vi "CONTROLE_COMPLETO_2808.vi"() -> ()   [LabVIEW 2017]
panel:
  in  "stop":bool
  out "CODIGO\nPEÇA":dbl
  out "POS_FUT":dbl
  out "POS_ATUAL":dbl
  out "DEPÓSITO":bool
  out "POSICIONAMENTO":bool
  out "TRANSPORTE":bool
  out "EM ESPERA":bool
  in  "RUN":bool
  in  "SENTIDO":bool
  in  "ESTEIRA":bool
  out "MANUAL":bool
  out "AUTOMÁTICO":bool
  in  "MAN":bool
  out "COD_S4 2":dbl
  in  "TAMANHO_S4 2":enum16{"PEQUENO", "MÉDIO", "GRANDE", "DEFAULT"}(ring)
  in  "COR_S4 2":enum16{"COR 3", "COR 2", "COR 1", "DEFAULT"}(ring)
  in  "MATERIAL_S4 2":enum16{"METÁLICO", "NÃO METÁLICO", "DEFAULT"}(ring)
  out "COD_S3 2":dbl
  in  "TAMANHO_S3 2":enum16{"PEQUENO", "MÉDIO", "GRANDE", "DEFAULT"}(ring)
  in  "COR_S3 2":enum16{"COR 3", "COR 2", "COR 1", "DEFAULT"}(ring)
  in  "MATERIAL_S3 2":enum16{"METÁLICO", "NÃO METÁLICO", "DEFAULT"}(ring)
  out "COD_S2 2":dbl
  in  "TAMANHO_S2 2":enum16{"PEQUENO", "MÉDIO", "GRANDE", "DEFAULT"}(ring)
  in  "COR_S2 2":enum16{"COR 3", "COR 2", "COR 1", "DEFAULT"}(ring)
  in  "MATERIAL_S2 2":enum16{"METÁLICO", "NÃO METÁLICO", "DEFAULT"}(ring)
  out "COD_S1 2":dbl
  in  "TAMANHO_S1 2":enum16{"PEQUENO", "MÉDIO", "GRANDE", "DEFAULT"}(ring)
  in  "COR_S1 2":enum16{"COR 3", "COR 2", "COR 1", "DEFAULT"}(ring)
  in  "MATERIAL_S1 2":enum16{"METÁLICO", "NÃO METÁLICO", "DEFAULT"}(ring)
  out "CONFIGURAÇÃO CONFLITANTE 2":bool
  out "PEÇA NÃO\nCONFIGURADA":bool
  out "ESTEIRA RUN":bool
  out "PEÇA NO\nSLOT":bool
  out "MATERIAL\nMETÁLICO":bool
  out "COR_3I 2":bool
  out "COR_2I 2":bool
  out "COR_1I 2":bool
  out "TAM_PI 2":bool
  out "TAM_MI 2":bool
  out "TAM_GI 2":bool
  out "PEÇA NA\nESTEIRA":bool
  out "ESQ 2":bool
  out "DIR 2":bool
  out "RUN":bool
  out "SLOT 8":bool
  out "SLOT 7":bool
  out "SLOT 6":bool
  out "SLOT 5":bool
  out "POS_4 2":bool
  out "POS_3 2":bool
  out "POS_2 2":bool
  out "POS_1 2":bool
  out "Numeric 2":i32
  out "Numeric":i32
  in  "RESET":bool
  out "COD_CT":dbl
  out "COD_MT":dbl
  out "COD_MC":dbl
  out "COD_T":dbl
  out "COD_C":dbl
  out "COD_M":dbl
  out "2":bool
  out "4":bool
  out "3":bool
  out "1":bool
  out "CONT_1":dbl
  # "MÓDULO"
  # "UNIVERSIDADE FEDERAL DE SÃO JOÃO DEL-REI\nCAMPUS ALTO PARAOPEBA - ENGENHARIA MECATRÔNICA"
  # "2808"
  # "LABORATÓRIO DE CONTROLE E AUTOMAÇÃO"
  # "MODO"
  # "CONTROLE MANUAL"
  # "CONFIGURAÇÃO DO SISTEMA DE SELEÇÃO"
  # "SLOT 1"
  # "SLOT 2"
  # "SLOT 3"
  # "SLOT 4"
  # "POSICIONADOR"
  # "MATERIAL"
  # "RUN"
  # "COR"
  # "CONTROLE AUTOMÁTICO"
  # "TAMANHO"
  # "CÓDIGO\nSLOT"
  # "SINÓPTICO SISTEMA DE CONTROLE, SELEÇÃO E TRANSPORTE DE PEÇAS"
  # "PEÇA GRANDE"
  # "COR 1"
  # "POSIÇÃO\nATUAL"
  # "COR 2"
  # "PEÇA MÉDIA"
  # "1"
  # "2"
  # "3"
  # "4"
  # "COR 3"
  # "PEÇA PEQUENA"
  # "ESQ"
  # "MOTOR POSICIONADOR"
  # "DIR"
  # "MOTOR\nESTEIRA"
  # "POSIÇÃO\nFUTURA"
  # "1"
  # "2"
  # "4"
  # "3"
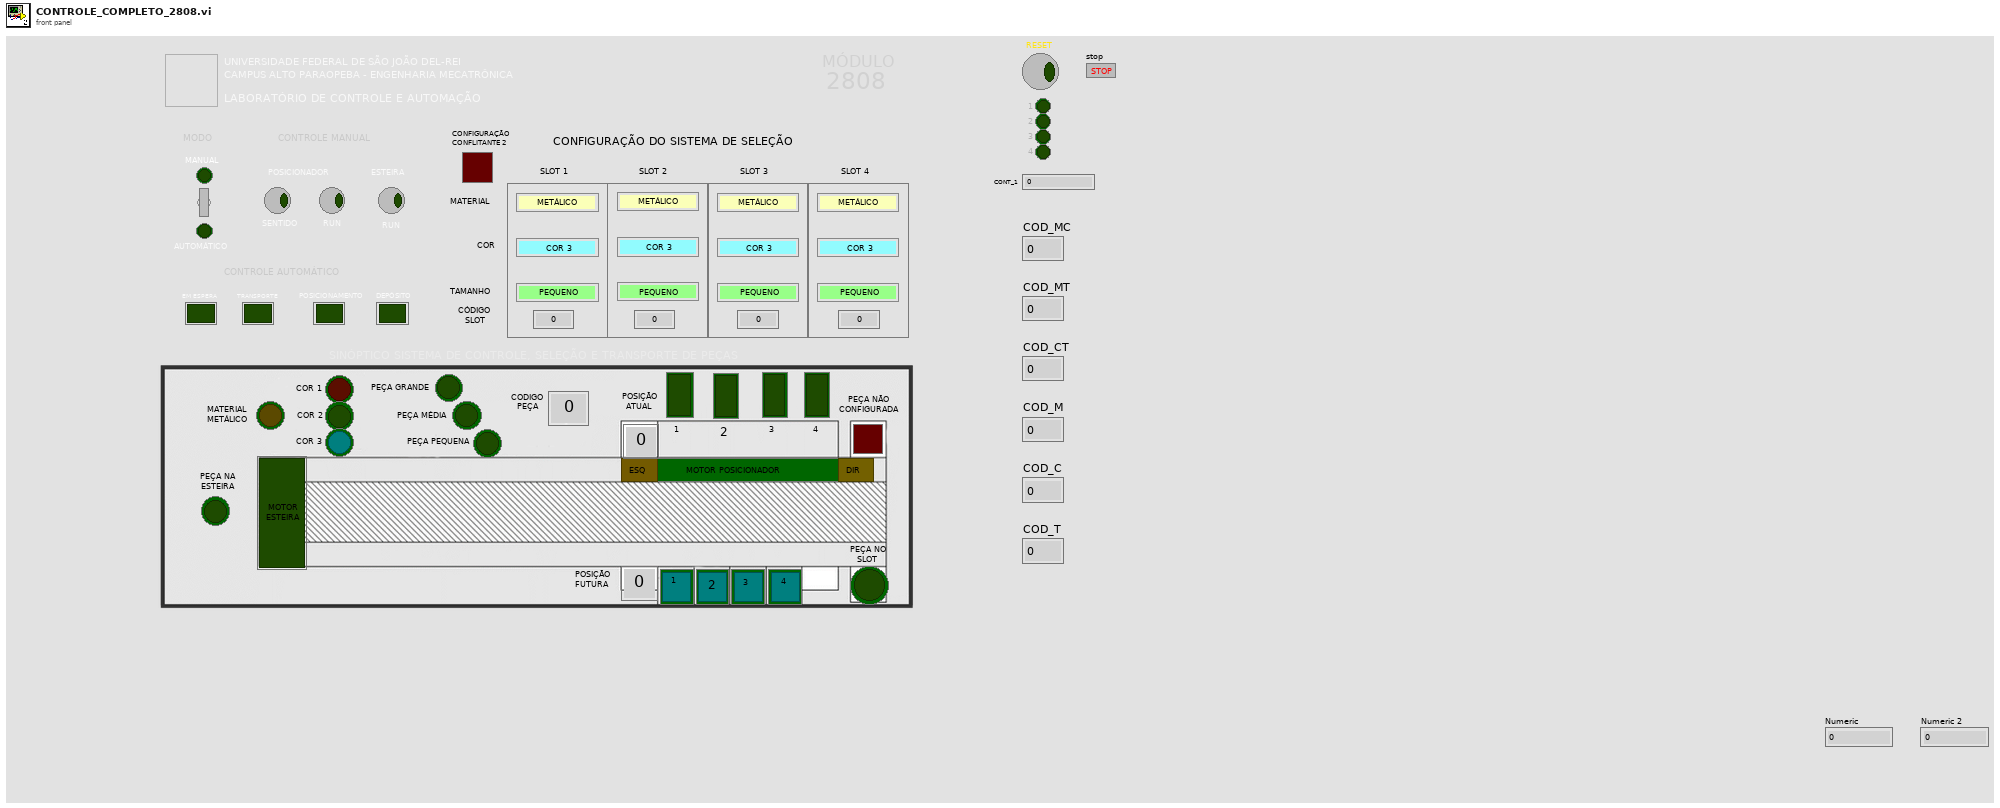
[diagram p1: front panel]
types:
  T1 = enum16{"DEPOSITO HASTE", "POSICIONAMENTO HASTE", "AQUISIÇÃO DE DADOS", "EM ESPERA"}
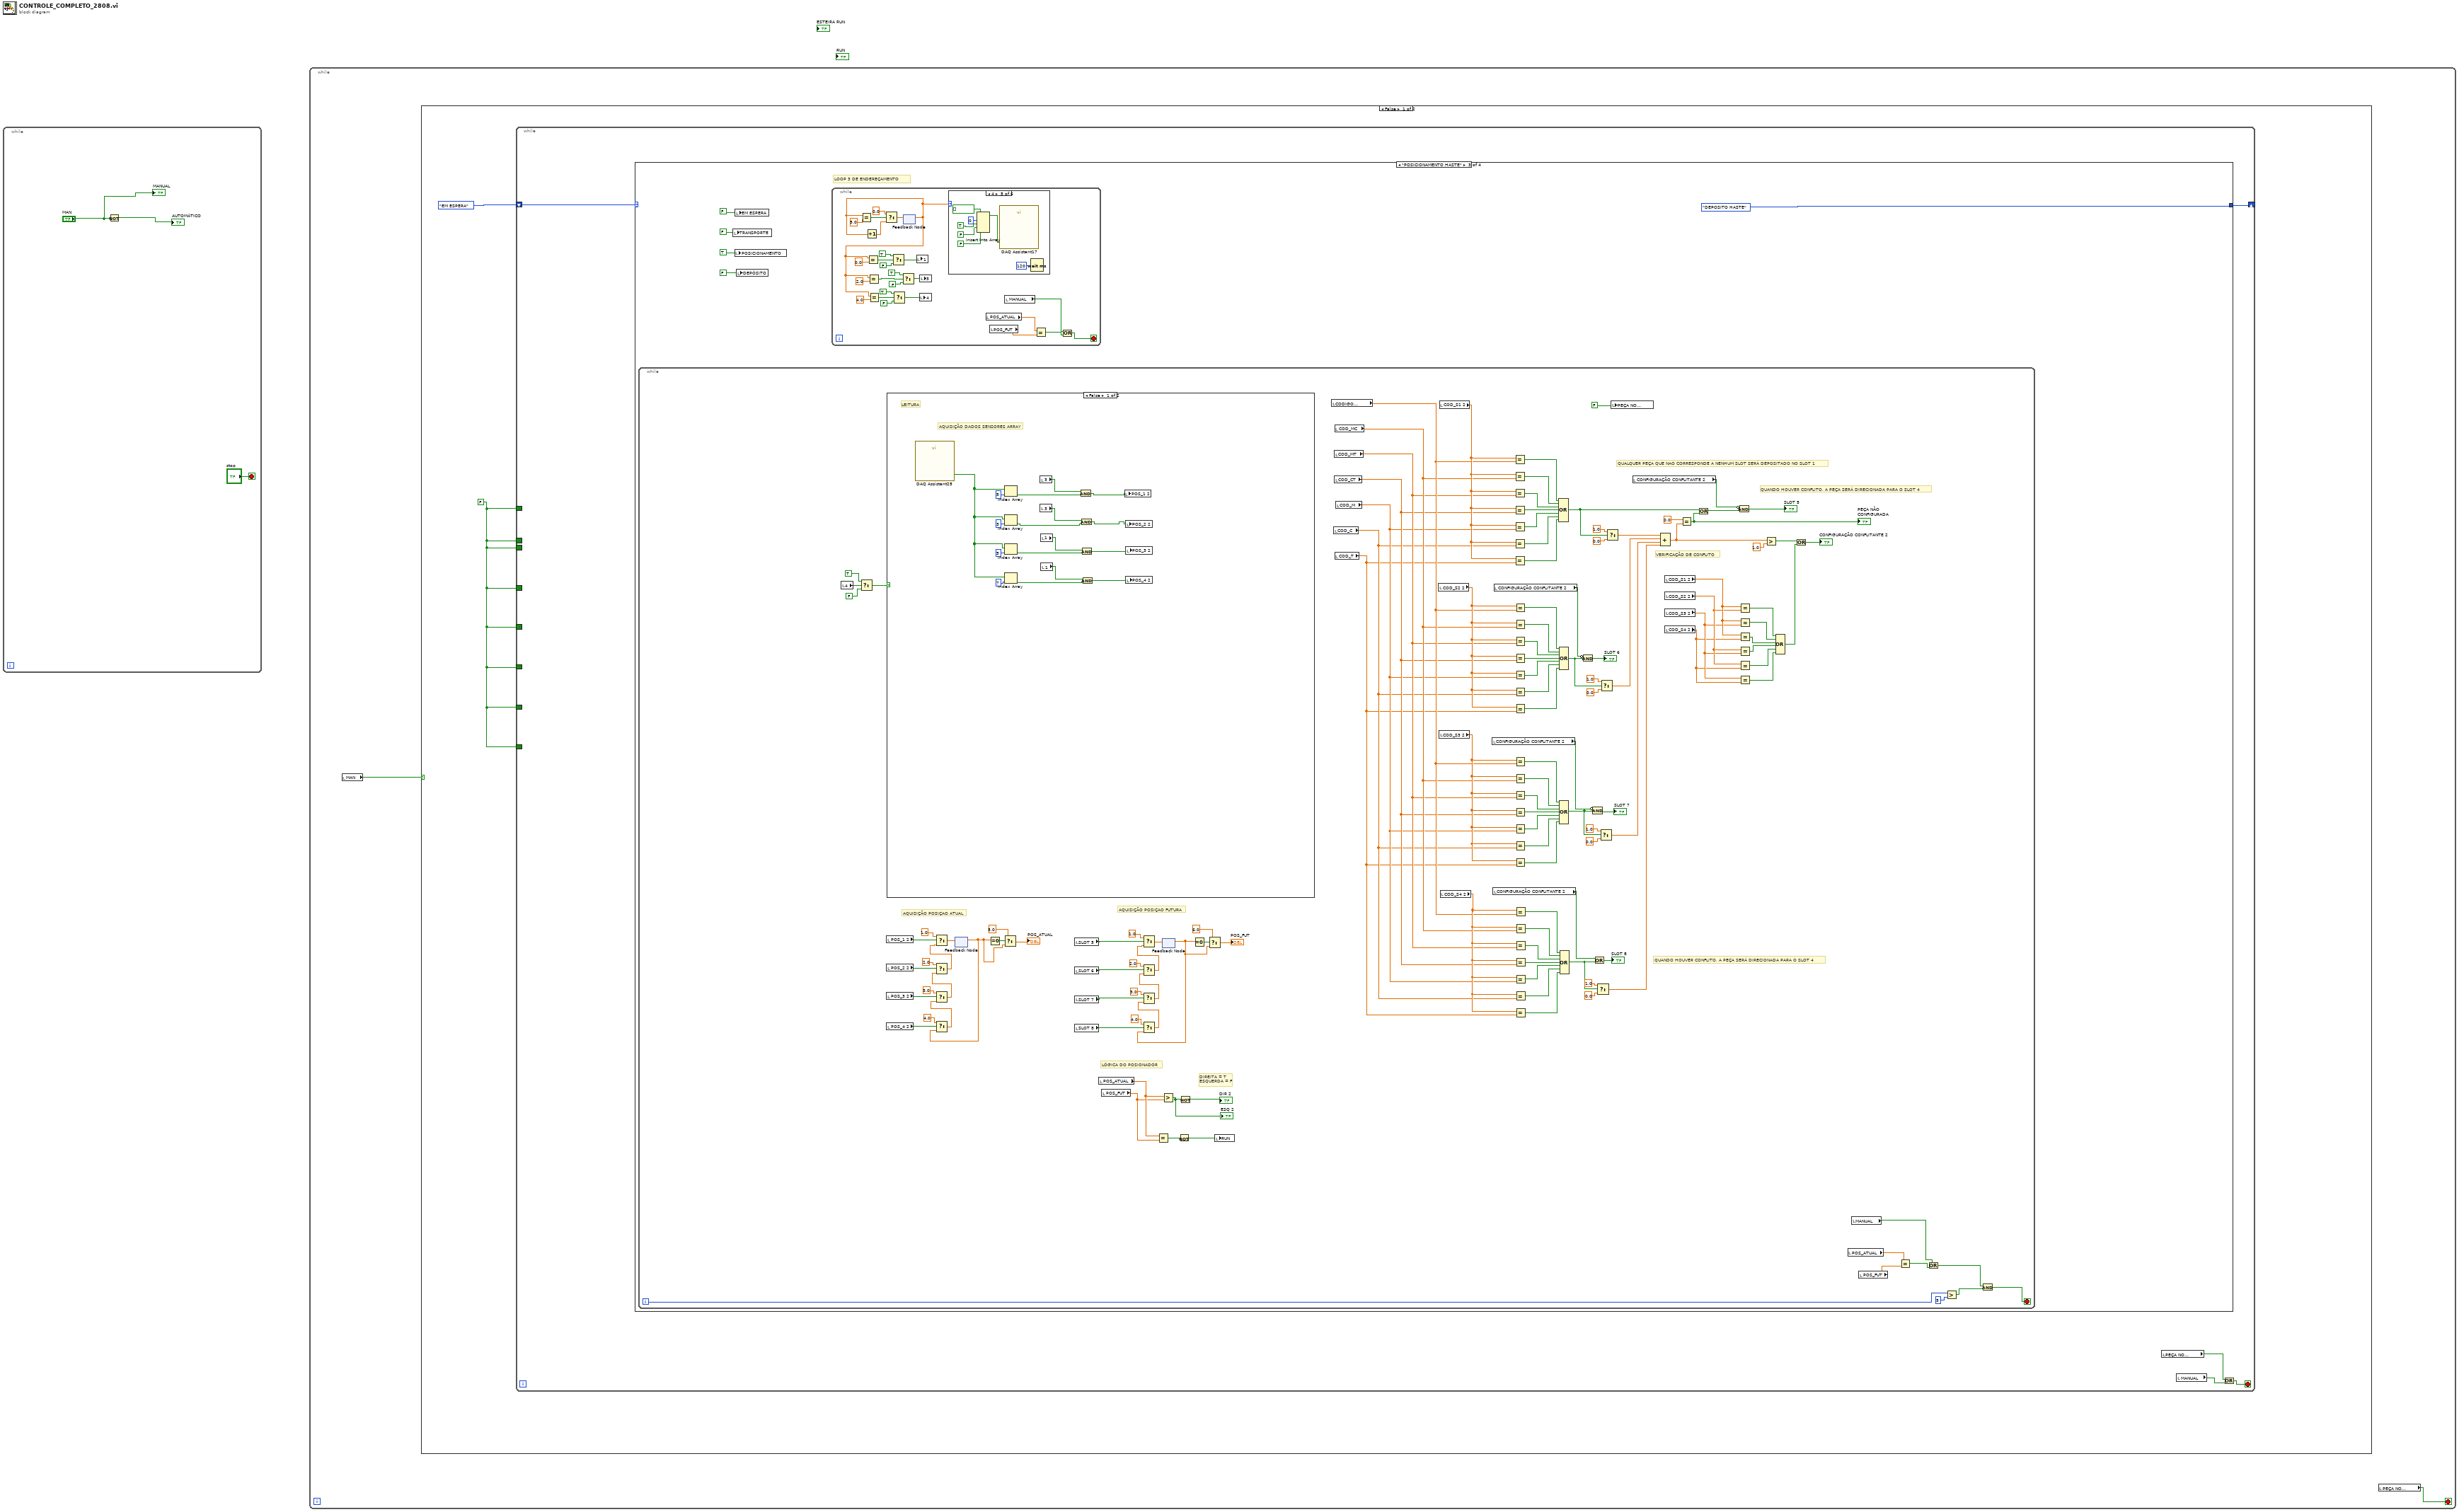
[diagram p0: block diagram]
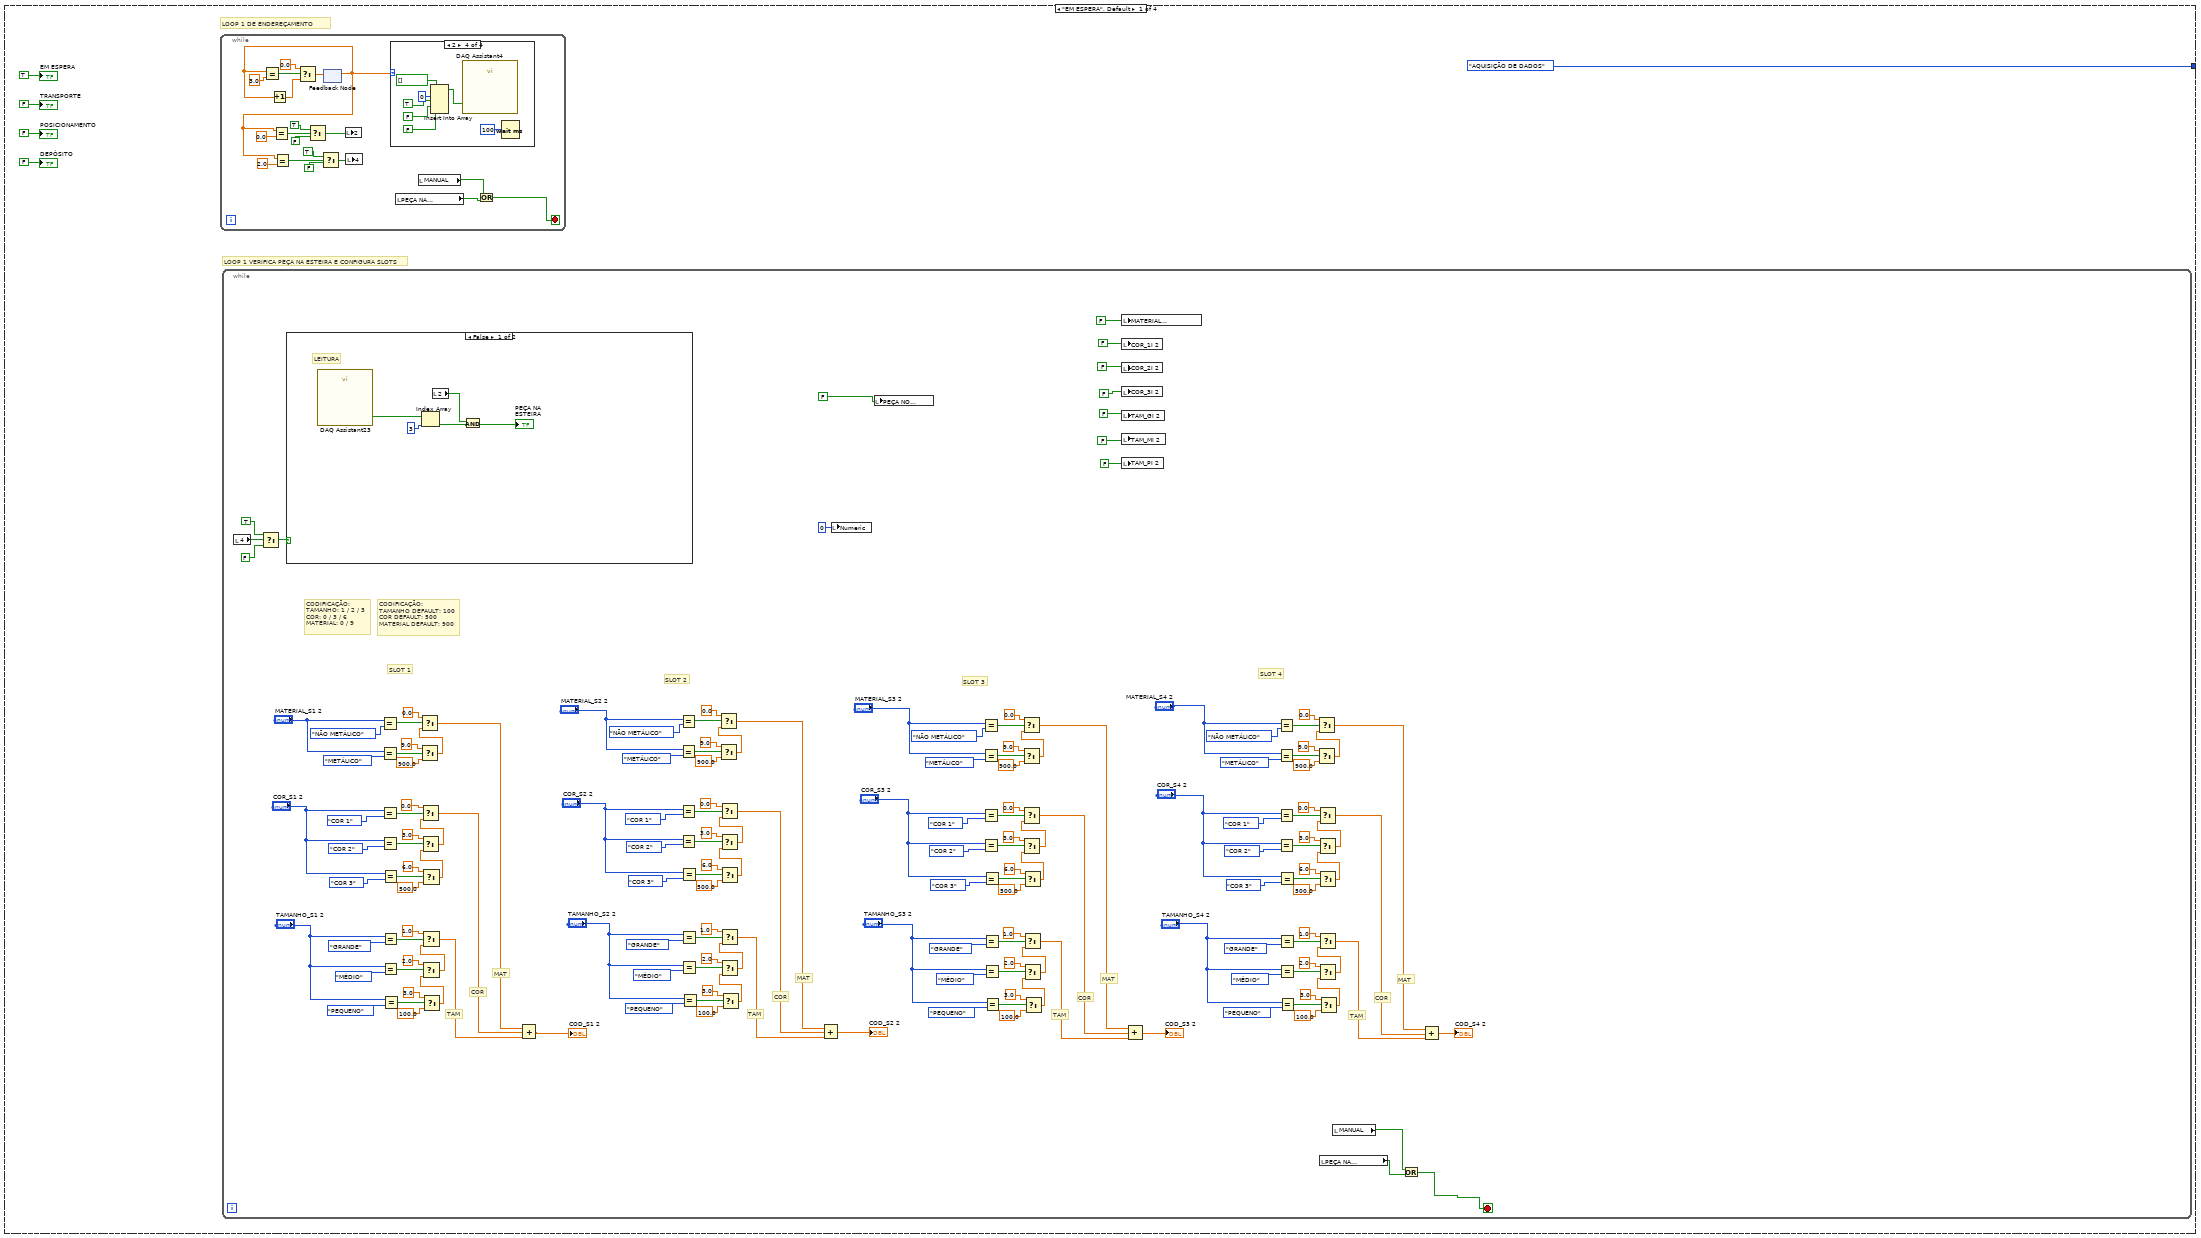
[diagram p2: hidden frame]
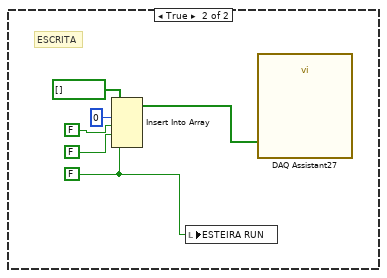
[diagram p3: hidden frame]
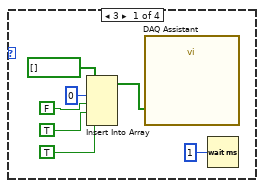
[diagram p4: hidden frame]
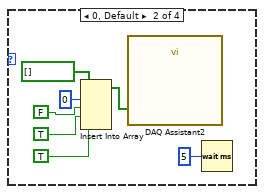
[diagram p5: hidden frame]
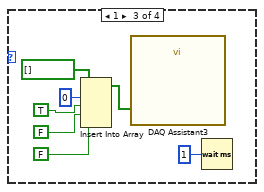
[diagram p6: hidden frame]
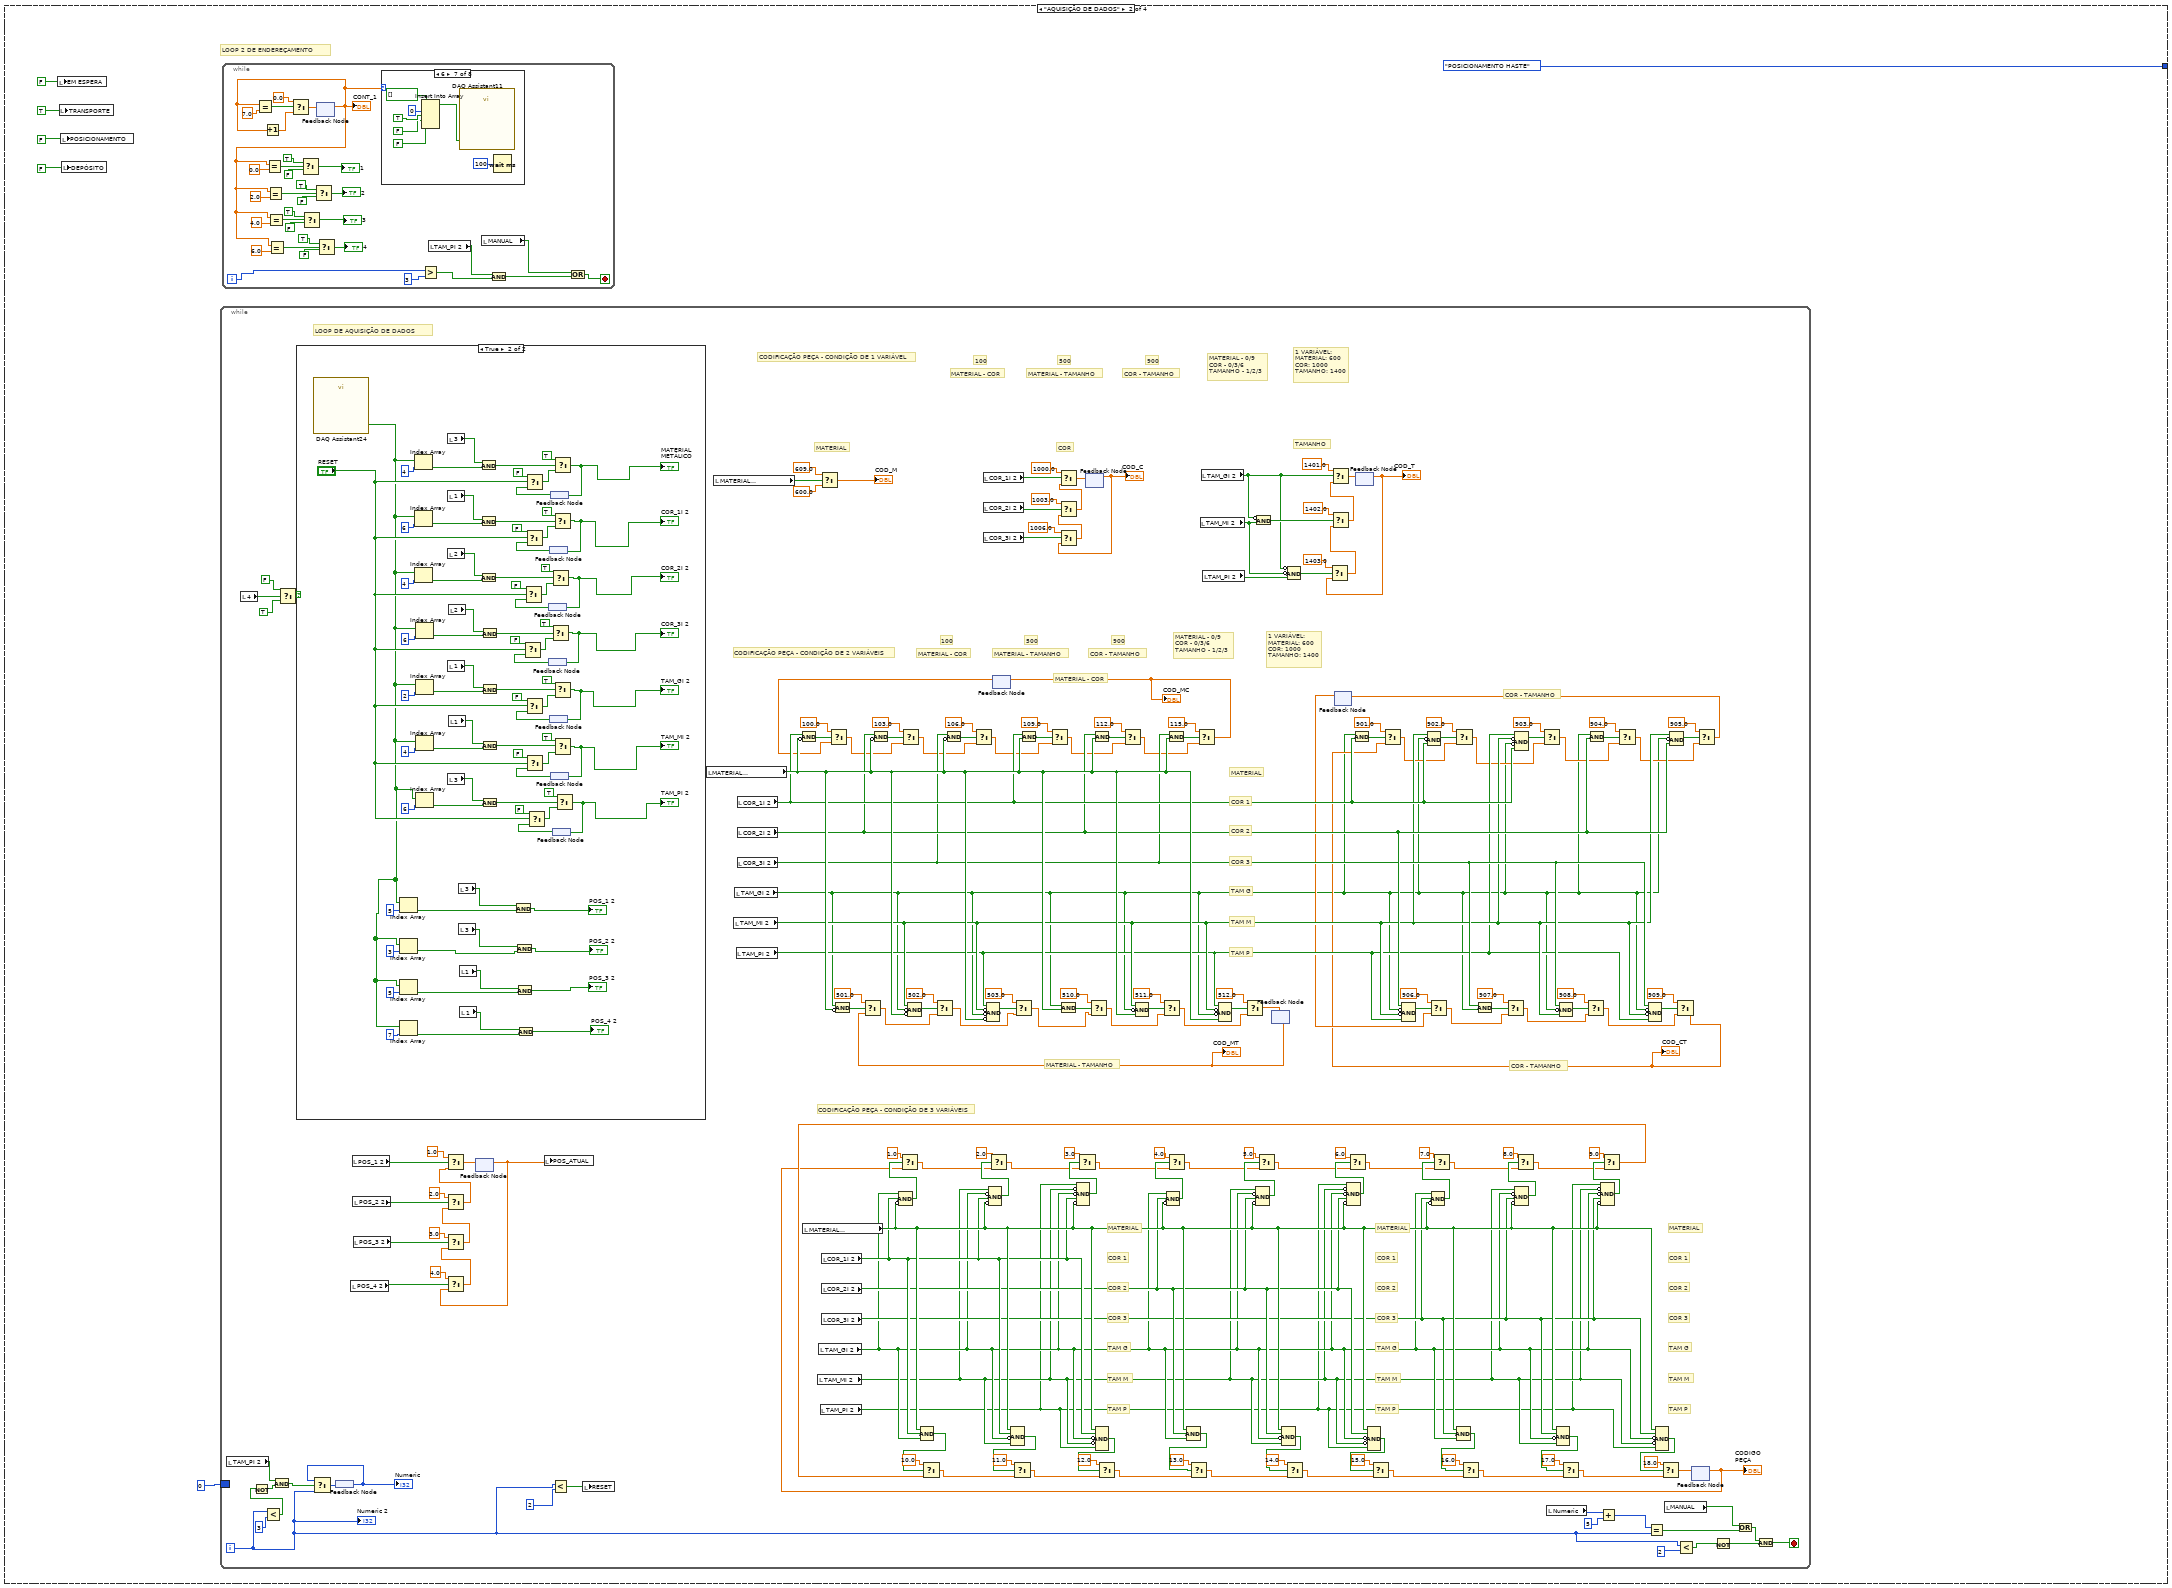
[diagram p7: hidden frame]
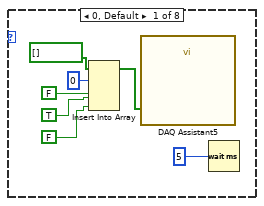
[diagram p8: hidden frame]
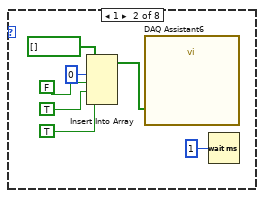
[diagram p9: hidden frame]
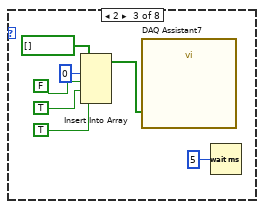
[diagram p10: hidden frame]
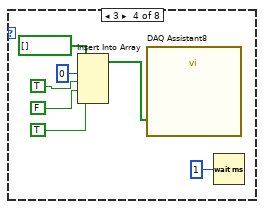
[diagram p11: hidden frame]
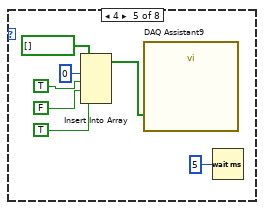
[diagram p12: hidden frame]
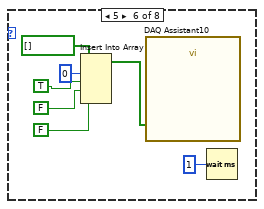
[diagram p13: hidden frame]
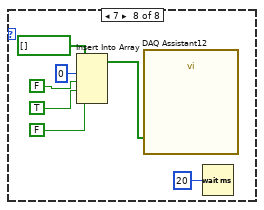
[diagram p14: hidden frame]
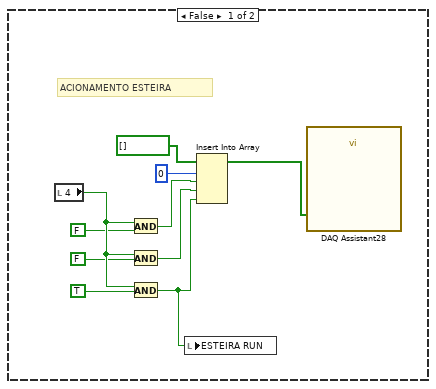
[diagram p15: hidden frame]
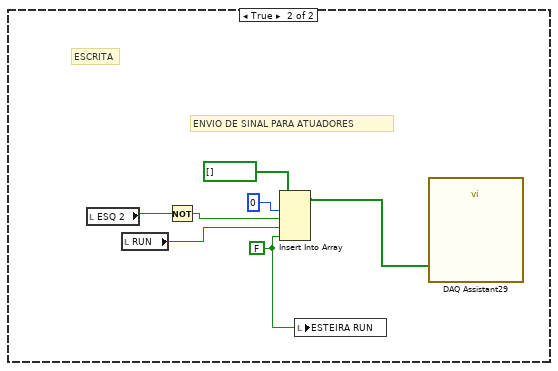
[diagram p16: hidden frame]
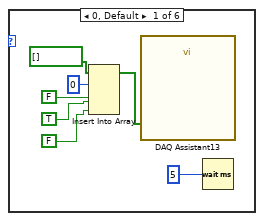
[diagram p17: hidden frame]
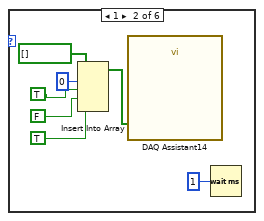
[diagram p18: hidden frame]
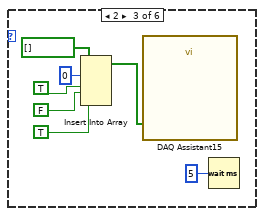
[diagram p19: hidden frame]
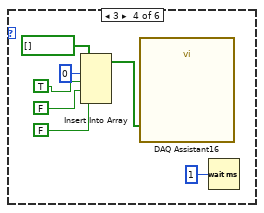
[diagram p20: hidden frame]
diagram:
  n1 = while {
    stop <- "stop" stop-if-true
    n2 = Not(x="MAN") -> (.not. x?=→"AUTOMÁTICO":bool)
    "MANUAL" <- "MAN"
  }
  n3 = while {
    stop <- w4 stop-if-true
    n4 = local read "MAN"() -> (w5:bool)
    n5 = case shown="False" w5 {
      frame False {
        w6 = FALSE
        n6 = while {
          shift-right: [w11] -> _
          shift-left: T1."EM ESPERA" -> [w12]
          border: w6 -> [_]
          border: w6 -> [_]
          border: w6 -> [_]
          border: w6 -> [_]
          border: w6 -> [_]
          border: w6 -> [_]
          border: w6 -> [_]
          border: w6 -> [_]
          stop <- w8 stop-if-true
          n7 = case shown="\"POSICIONAMENTO HASTE\"" w12 {
            tunnel: [T1."AQUISIÇÃO DE DADOS" T1."POSICIONAMENTO HASTE" T1."DEPOSITO HASTE" T1."EM ESPERA"] -> w11
            frame "EM ESPERA", Default {
              # "LOOP 1 VERIFICA PEÇA NA ESTEIRA E CONFIGURA SLOTS"
              # "LOOP 1 DE ENDEREÇAMENTO"
              n8 = while {
                stop <- w201 stop-if-true
                n9 = feedback #1() -> (w206:dbl)  [unwired: 1 in]
                n10 = Equal?(x=w206, y=3.0) -> (x = y?=w219:bool)
                n11 = Increment(x=w206) -> (x+1=w216:dbl)
                n12 = Equal?(x=w206, y=0.0) -> (x = y?=w212:bool)
                n13 = Equal?(x=w206, y=2.0) -> (x = y?=w207:bool)
                n14 = Select(t=0.0, s=w219, f=w216) -> (s? t:f=w218:dbl)
                n15 = Select(t=TRUE, s=w212, f=FALSE) -> (s? t:f=w205:bool)
                n16 = Select(t=TRUE, s=w207, f=FALSE) -> (s? t:f=w204:bool)
                n17 = feedback-in #1(w218) -> ()
                n18 = local write "2"(w205) -> ()
                n19 = local write "4"(w204) -> ()
                n20 = case shown="2" w206 {
                  frame 3 {
                    n21 = Insert Into Array(array=bool[] [], index=0, new element #1=FALSE, new element #2=TRUE, new element #3=TRUE) -> (w220:bool[])
                    n22 = call "DAQ Assistant"("data"=w220) -> ()  [unwired: 17 in, 2 out]
                    n23 = Wait (ms)(milliseconds to wait=u32 1) -> ()  [unwired: 1 out]
                  }
                  frame 0, Default {
                    n24 = Insert Into Array(array=bool[] [], index=0, new element #1=FALSE, new element #2=TRUE, new element #3=TRUE) -> (w227:bool[])
                    n25 = call "DAQ Assistant2"("data"=w227) -> ()  [unwired: 17 in, 2 out]
                    n26 = Wait (ms)(milliseconds to wait=u32 5) -> ()  [unwired: 1 out]
                  }
                  frame 1 {
                    n27 = Insert Into Array(array=bool[] [], index=0, new element #1=TRUE, new element #2=FALSE, new element #3=FALSE) -> (w234:bool[])
                    n28 = call "DAQ Assistant3"("data"=w234) -> ()  [unwired: 17 in, 2 out]
                    n29 = Wait (ms)(milliseconds to wait=u32 1) -> ()  [unwired: 1 out]
                  }
                  frame 2 {
                    n30 = Insert Into Array(array=bool[] [], index=0, new element #1=TRUE, new element #2=FALSE, new element #3=FALSE) -> (w241:bool[])
                    n31 = call "DAQ Assistant4"("data"=w241) -> ()  [unwired: 17 in, 2 out]
                    n32 = Wait (ms)(milliseconds to wait=u32 100) -> ()  [unwired: 1 out]
                  }
                }
                n33 = local read "PEÇA NA\nESTEIRA"() -> (w203:bool)
                n34 = local read "MANUAL"() -> (w202:bool)
                n35 = Or(x=w202, y=w203) -> (x .or. y?=w201:bool)
              }
              n36 = while {
                stop <- w42 stop-if-true
                # "COR"
                # "MAT"
                # "TAM"
                # "COR"
                # "MAT"
                # "TAM"
                # "COR"
                # "MAT"
                # "TAM"
                # "TAM"
                # "COR"
                # "MAT"
                # "CODIFICAÇÃO:\nTAMANHO DEFAULT: 100\nCOR DEFAULT: 500\nMATERIAL DEFAULT: 900"
                # "CODIFICAÇÃO:\nTAMANHO: 1 / 2 / 3\nCOR: 0 / 3 / 6\nMATERIAL: 0 / 9"
                # "SLOT 4"
                # "SLOT 3"
                # "SLOT 2"
                # "SLOT 1"
                n37 = local read "4"() -> (w189:bool)
                n38 = Select(t=TRUE, s=w189, f=FALSE) -> (s? t:f=w186:bool)
                n39 = case shown="False" w186 {
                  frame False {
                    # "LEITURA"
                    n40 = call "DAQ Assistant23"() -> ("data"=w191:bool[])  [unwired: 17 in, 2 out]
                    n41 = Index Array(array=w191, index=3) -> (element=w192:bool)
                    n42 = local read "2"() -> (w194:bool)
                    n43 = And(x=w194, y=w192) -> (x .and. y?=→"PEÇA NA\nESTEIRA":bool)
                  }
                  frame True {
                    w196 = FALSE
                    # "ESCRITA"
                    n44 = Insert Into Array(array=bool[] [], index=0, new element #1=FALSE, new element #2=FALSE, new element #3=w196) -> (w195:bool[])
                    n45 = local write "ESTEIRA RUN"(w196) -> ()
                    n46 = call "DAQ Assistant27"("data"=w195) -> ()  [unwired: 17 in, 2 out]
                  }
                }
                n47 = Equal?(x="MATERIAL_S1 2", y=enum16{"METÁLICO", "NÃO METÁLICO", "DEFAULT"}."NÃO METÁLICO") -> (x = y?=w185:bool)
                n48 = Equal?(x="MATERIAL_S1 2", y=enum16{"METÁLICO", "NÃO METÁLICO", "DEFAULT"}."METÁLICO") -> (x = y?=w181:bool)
                n49 = Equal?(x="COR_S1 2", y=enum16{"COR 3", "COR 2", "COR 1", "DEFAULT"}."COR 1") -> (x = y?=w177:bool)
                n50 = Equal?(x="COR_S1 2", y=enum16{"COR 3", "COR 2", "COR 1", "DEFAULT"}."COR 2") -> (x = y?=w176:bool)
                n51 = Equal?(x="COR_S1 2", y=enum16{"COR 3", "COR 2", "COR 1", "DEFAULT"}."COR 3") -> (x = y?=w175:bool)
                n52 = Equal?(x="TAMANHO_S1 2", y=enum16{"PEQUENO", "MÉDIO", "GRANDE", "DEFAULT"}."GRANDE") -> (x = y?=w165:bool)
                n53 = Equal?(x="TAMANHO_S1 2", y=enum16{"PEQUENO", "MÉDIO", "GRANDE", "DEFAULT"}."MÉDIO") -> (x = y?=w164:bool)
                n54 = Equal?(x="TAMANHO_S1 2", y=enum16{"PEQUENO", "MÉDIO", "GRANDE", "DEFAULT"}."PEQUENO") -> (x = y?=w163:bool)
                n55 = Select(t=9.0, s=w181, f=900.0) -> (s? t:f=w178:dbl)
                n56 = Select(t=0.0, s=w185, f=w178) -> (s? t:f=w57:dbl)
                n57 = Select(t=6.0, s=w175, f=500.0) -> (s? t:f=w167:dbl)
                n58 = Select(t=3.0, s=w176, f=w167) -> (s? t:f=w166:dbl)
                n59 = Select(t=0.0, s=w177, f=w166) -> (s? t:f=w56:dbl)
                n60 = Select(t=3.0, s=w163, f=100.0) -> (s? t:f=w158:dbl)
                n61 = Select(t=2.0, s=w164, f=w158) -> (s? t:f=w157:dbl)
                n62 = Select(t=1.0, s=w165, f=w157) -> (s? t:f=w55:dbl)
                n63 = Compound Arithmetic op=ADD(w57, w56, w55) -> (→"COD_S1 2":dbl)
                n64 = Equal?(x="MATERIAL_S2 2", y=enum16{"METÁLICO", "NÃO METÁLICO", "DEFAULT"}."NÃO METÁLICO") -> (x = y?=w153:bool)
                n65 = Equal?(x="MATERIAL_S2 2", y=enum16{"METÁLICO", "NÃO METÁLICO", "DEFAULT"}."METÁLICO") -> (x = y?=w149:bool)
                n66 = Equal?(x="COR_S2 2", y=enum16{"COR 3", "COR 2", "COR 1", "DEFAULT"}."COR 1") -> (x = y?=w145:bool)
                n67 = Equal?(x="COR_S2 2", y=enum16{"COR 3", "COR 2", "COR 1", "DEFAULT"}."COR 2") -> (x = y?=w144:bool)
                n68 = Equal?(x="COR_S2 2", y=enum16{"COR 3", "COR 2", "COR 1", "DEFAULT"}."COR 3") -> (x = y?=w143:bool)
                n69 = Equal?(x="TAMANHO_S2 2", y=enum16{"PEQUENO", "MÉDIO", "GRANDE", "DEFAULT"}."GRANDE") -> (x = y?=w133:bool)
                n70 = Equal?(x="TAMANHO_S2 2", y=enum16{"PEQUENO", "MÉDIO", "GRANDE", "DEFAULT"}."MÉDIO") -> (x = y?=w132:bool)
                n71 = Equal?(x="TAMANHO_S2 2", y=enum16{"PEQUENO", "MÉDIO", "GRANDE", "DEFAULT"}."PEQUENO") -> (x = y?=w131:bool)
                n72 = Select(t=9.0, s=w149, f=900.0) -> (s? t:f=w146:dbl)
                n73 = Select(t=0.0, s=w153, f=w146) -> (s? t:f=w52:dbl)
                n74 = Select(t=6.0, s=w143, f=500.0) -> (s? t:f=w135:dbl)
                n75 = Select(t=3.0, s=w144, f=w135) -> (s? t:f=w134:dbl)
                n76 = Select(t=0.0, s=w145, f=w134) -> (s? t:f=w53:dbl)
                n77 = Select(t=3.0, s=w131, f=100.0) -> (s? t:f=w126:dbl)
                n78 = Select(t=2.0, s=w132, f=w126) -> (s? t:f=w125:dbl)
                n79 = Select(t=1.0, s=w133, f=w125) -> (s? t:f=w54:dbl)
                n80 = Compound Arithmetic op=ADD(w52, w53, w54) -> (→"COD_S2 2":dbl)
                n81 = local write "Numeric"(0 ("Numeric")) -> ()
                n82 = local write "PEÇA NO\nSLOT"(FALSE ("PDS_I")) -> ()
                n83 = Equal?(x="MATERIAL_S3 2", y=enum16{"METÁLICO", "NÃO METÁLICO", "DEFAULT"}."NÃO METÁLICO") -> (x = y?=w121:bool)
                n84 = Equal?(x="MATERIAL_S3 2", y=enum16{"METÁLICO", "NÃO METÁLICO", "DEFAULT"}."METÁLICO") -> (x = y?=w117:bool)
                n85 = Equal?(x="COR_S3 2", y=enum16{"COR 3", "COR 2", "COR 1", "DEFAULT"}."COR 1") -> (x = y?=w113:bool)
                n86 = Equal?(x="COR_S3 2", y=enum16{"COR 3", "COR 2", "COR 1", "DEFAULT"}."COR 2") -> (x = y?=w112:bool)
                n87 = Equal?(x="COR_S3 2", y=enum16{"COR 3", "COR 2", "COR 1", "DEFAULT"}."COR 3") -> (x = y?=w111:bool)
                n88 = Equal?(x="TAMANHO_S3 2", y=enum16{"PEQUENO", "MÉDIO", "GRANDE", "DEFAULT"}."GRANDE") -> (x = y?=w101:bool)
                n89 = Equal?(x="TAMANHO_S3 2", y=enum16{"PEQUENO", "MÉDIO", "GRANDE", "DEFAULT"}."MÉDIO") -> (x = y?=w100:bool)
                n90 = Equal?(x="TAMANHO_S3 2", y=enum16{"PEQUENO", "MÉDIO", "GRANDE", "DEFAULT"}."PEQUENO") -> (x = y?=w99:bool)
                n91 = Select(t=9.0, s=w117, f=900.0) -> (s? t:f=w114:dbl)
                n92 = Select(t=0.0, s=w121, f=w114) -> (s? t:f=w49:dbl)
                n93 = Select(t=6.0, s=w111, f=500.0) -> (s? t:f=w103:dbl)
                n94 = Select(t=3.0, s=w112, f=w103) -> (s? t:f=w102:dbl)
                n95 = Select(t=0.0, s=w113, f=w102) -> (s? t:f=w50:dbl)
                n96 = Select(t=3.0, s=w99, f=100.0) -> (s? t:f=w94:dbl)
                n97 = Select(t=2.0, s=w100, f=w94) -> (s? t:f=w93:dbl)
                n98 = Select(t=1.0, s=w101, f=w93) -> (s? t:f=w51:dbl)
                n99 = local write "MATERIAL\nMETÁLICO"(FALSE) -> ()
                n100 = local write "COR_1I 2"(FALSE) -> ()
                n101 = local write "COR_2I 2"(FALSE) -> ()
                n102 = local write "COR_3I 2"(FALSE) -> ()
                n103 = local write "TAM_GI 2"(FALSE) -> ()
                n104 = local write "TAM_MI 2"(FALSE) -> ()
                n105 = local write "TAM_PI 2"(FALSE) -> ()
                n106 = Compound Arithmetic op=ADD(w49, w50, w51) -> (→"COD_S3 2":dbl)
                n107 = Equal?(x="MATERIAL_S4 2", y=enum16{"METÁLICO", "NÃO METÁLICO", "DEFAULT"}."NÃO METÁLICO") -> (x = y?=w89:bool)
                n108 = Equal?(x="MATERIAL_S4 2", y=enum16{"METÁLICO", "NÃO METÁLICO", "DEFAULT"}."METÁLICO") -> (x = y?=w85:bool)
                n109 = Equal?(x="COR_S4 2", y=enum16{"COR 3", "COR 2", "COR 1", "DEFAULT"}."COR 1") -> (x = y?=w81:bool)
                n110 = Equal?(x="COR_S4 2", y=enum16{"COR 3", "COR 2", "COR 1", "DEFAULT"}."COR 2") -> (x = y?=w80:bool)
                n111 = Equal?(x="COR_S4 2", y=enum16{"COR 3", "COR 2", "COR 1", "DEFAULT"}."COR 3") -> (x = y?=w79:bool)
                n112 = Equal?(x="TAMANHO_S4 2", y=enum16{"PEQUENO", "MÉDIO", "GRANDE", "DEFAULT"}."GRANDE") -> (x = y?=w69:bool)
                n113 = Equal?(x="TAMANHO_S4 2", y=enum16{"PEQUENO", "MÉDIO", "GRANDE", "DEFAULT"}."MÉDIO") -> (x = y?=w68:bool)
                n114 = Equal?(x="TAMANHO_S4 2", y=enum16{"PEQUENO", "MÉDIO", "GRANDE", "DEFAULT"}."PEQUENO") -> (x = y?=w67:bool)
                n115 = Select(t=9.0, s=w85, f=900.0) -> (s? t:f=w82:dbl)
                n116 = Select(t=0.0, s=w89, f=w82) -> (s? t:f=w46:dbl)
                n117 = Select(t=6.0, s=w79, f=500.0) -> (s? t:f=w71:dbl)
                n118 = Select(t=3.0, s=w80, f=w71) -> (s? t:f=w70:dbl)
                n119 = Select(t=0.0, s=w81, f=w70) -> (s? t:f=w47:dbl)
                n120 = Select(t=3.0, s=w67, f=100.0) -> (s? t:f=w62:dbl)
                n121 = Select(t=2.0, s=w68, f=w62) -> (s? t:f=w61:dbl)
                n122 = Select(t=1.0, s=w69, f=w61) -> (s? t:f=w48:dbl)
                n123 = local read "PEÇA NA\nESTEIRA"() -> (w45:bool)
                n124 = local read "MANUAL"() -> (w44:bool)
                n125 = Or(x=w44, y=w45) -> (x .or. y?=w42:bool)
                n126 = Compound Arithmetic op=ADD(w46, w47, w48) -> (→"COD_S4 2":dbl)
              }
              "TRANSPORTE" <- FALSE
              "POSICIONAMENTO" <- FALSE
              "DEPÓSITO" <- FALSE
              "EM ESPERA" <- TRUE
            }
            frame "AQUISIÇÃO DE DADOS" {
              # "LOOP 2 DE ENDEREÇAMENTO"
              n127 = local write "EM ESPERA"(FALSE) -> ()
              n128 = local write "TRANSPORTE"(TRUE) -> ()
              n129 = local write "POSICIONAMENTO"(FALSE) -> ()
              n130 = local write "DEPÓSITO"(FALSE) -> ()
              n131 = while {
                border: 0 -> [_]
                i -> [w348]
                stop <- w352 stop-if-true
                # "CODIFICAÇÃO PEÇA - CONDIÇÃO DE 3 VARIÁVEIS"
                # "TAM P"
                # "TAM M"
                # "TAM G"
                # "COR 3"
                # "COR 2"
                # "COR 1"
                # "MATERIAL"
                # "TAM P"
                # "TAM M"
                # "TAM G"
                # "COR 3"
                # "COR 2"
                # "COR 1"
                # "MATERIAL"
                # "TAM P"
                # "TAM M"
                # "TAM G"
                # "COR 3"
                # "COR 2"
                # "COR 1"
                # "MATERIAL"
                # "1 VARIÁVEL:\nMATERIAL: 600\nCOR: 1000\nTAMANHO: 1400"
                # "COR - TAMANHO"
                # "COR - TAMANHO"
                # "MATERIAL - TAMANHO"
                # "MATERIAL - COR"
                # "MATERIAL - 0/9\nCOR - 0/3/6\nTAMANHO - 1/2/3"
                # "900"
                # "500"
                # "100"
                # "COR - TAMANHO"
                # "MATERIAL - TAMANHO"
                # "MATERIAL - COR"
                # "CODIFICAÇÃO PEÇA - CONDIÇÃO DE 2 VARIÁVEIS"
                # "TAM P"
                # "TAM M"
                # "TAM G"
                # "COR 3"
                # "COR 2"
                # "COR 1"
                # "MATERIAL"
                # "TAMANHO"
                # "COR"
                # "1 VARIÁVEL:\nMATERIAL: 600\nCOR: 1000\nTAMANHO: 1400"
                # "MATERIAL"
                # "MATERIAL - 0/9\nCOR - 0/3/6\nTAMANHO - 1/2/3"
                # "900"
                # "500"
                # "100"
                # "COR - TAMANHO"
                # "MATERIAL - TAMANHO"
                # "MATERIAL - COR"
                # "CODIFICAÇÃO PEÇA - CONDIÇÃO DE 1 VARIÁVEL"
                # "LOOP DE AQUISIÇÃO DE DADOS"
                n132 = local read "TAM_PI 2"() -> (w344:bool)
                n133 = local read "4"() -> (w540:bool)
                n134 = Less?(x=w348, y=3) -> (x < y?=w345:bool)
                n135 = Not(x=w345) -> (.not. x?=w346:bool)
                n136 = And(x=w344, y=w346) -> (x .and. y?=w343:bool)
                n137 = Select(t=FALSE, s=w540, f=TRUE) -> (s? t:f=w539:bool)
                n138 = case shown="True" w539 {
                  frame False {
                    # "ACIONAMENTO ESTEIRA"
                    n139 = local read "4"() -> (w550:bool)
                    n140 = And(x=w550, y=FALSE) -> (x .and. y?=w549:bool)
                    n141 = And(x=w550, y=FALSE) -> (x .and. y?=w548:bool)
                    n142 = And(x=w550, y=TRUE) -> (x .and. y?=w542:bool)
                    n143 = local write "ESTEIRA RUN"(w542) -> ()
                    n144 = Insert Into Array(array=bool[] [], index=0, new element #1=w549, new element #2=w548, new element #3=w542) -> (w541:bool[])
                    n145 = call "DAQ Assistant28"("data"=w541) -> ()  [unwired: 17 in, 2 out]
                  }
                  frame True {
                    n146 = call "DAQ Assistant24"() -> ("data"=w562:bool[])  [unwired: 17 in, 2 out]
                    n147 = Index Array(array=w562, index=5) -> (element=w566:bool)
                    n148 = Index Array(array=w562, index=3) -> (element=w565:bool)
                    n149 = Index Array(array=w562, index=5) -> (element=w564:bool)
                    n150 = Index Array(array=w562, index=7) -> (element=w563:bool)
                    n151 = Index Array(array=w562, index=4) -> (element=w577:bool)
                    n152 = Index Array(array=w562, index=6) -> (element=w576:bool)
                    n153 = Index Array(array=w562, index=4) -> (element=w575:bool)
                    n154 = Index Array(array=w562, index=6) -> (element=w574:bool)
                    n155 = Index Array(array=w562, index=2) -> (element=w573:bool)
                    n156 = Index Array(array=w562, index=4) -> (element=w572:bool)
                    n157 = Index Array(array=w562, index=6) -> (element=w571:bool)
                    n158 = local read "3"() -> (w596:bool)
                    n159 = local read "1"() -> (w595:bool)
                    n160 = local read "2"() -> (w594:bool)
                    n161 = local read "1"() -> (w592:bool)
                    n162 = local read "3"() -> (w590:bool)
                    n163 = local read "2"() -> (w593:bool)
                    n164 = local read "1"() -> (w591:bool)
                    n165 = local read "3"() -> (w589:bool)
                    n166 = local read "3"() -> (w588:bool)
                    n167 = local read "1"() -> (w587:bool)
                    n168 = local read "1"() -> (w586:bool)
                    n169 = And(x=w596, y=w577) -> (x .and. y?=w603:bool)
                    n170 = And(x=w595, y=w576) -> (x .and. y?=w602:bool)
                    n171 = And(x=w594, y=w575) -> (x .and. y?=w601:bool)
                    n172 = And(x=w593, y=w574) -> (x .and. y?=w600:bool)
                    n173 = And(x=w592, y=w573) -> (x .and. y?=w599:bool)
                    n174 = And(x=w591, y=w572) -> (x .and. y?=w598:bool)
                    n175 = And(x=w590, y=w571) -> (x .and. y?=w597:bool)
                    n176 = And(x=w589, y=w566) -> (x .and. y?=→"POS_1 2":bool)
                    n177 = And(x=w588, y=w565) -> (x .and. y?=→"POS_2 2":bool)
                    n178 = And(x=w587, y=w564) -> (x .and. y?=→"POS_3 2":bool)
                    n179 = And(x=w586, y=w563) -> (x .and. y?=→"POS_4 2":bool)
                    n180 = feedback #2() -> (w616:bool)
                    n181 = Select(t=FALSE, s="RESET", f=w616) -> (s? t:f=w617:bool)
                    n182 = feedback #3() -> (w620:bool)
                    n183 = Select(t=FALSE, s="RESET", f=w620) -> (s? t:f=w621:bool)
                    n184 = feedback #4() -> (w624:bool)
                    n185 = Select(t=FALSE, s="RESET", f=w624) -> (s? t:f=w625:bool)
                    n186 = feedback #5() -> (w612:bool)
                    n187 = Select(t=FALSE, s="RESET", f=w612) -> (s? t:f=w613:bool)
                    n188 = feedback #6() -> (w628:bool)
                    n189 = Select(t=FALSE, s="RESET", f=w628) -> (s? t:f=w629:bool)
                    n190 = feedback #7() -> (w608:bool)
                    n191 = Select(t=FALSE, s="RESET", f=w608) -> (s? t:f=w609:bool)
                    n192 = Select(t=TRUE, s=w600, f=w617) -> (s? t:f=w558:bool)
                    "COR_3I 2" <- w558
                    n193 = feedback-in #2(w558) -> ()
                    n194 = Select(t=TRUE, s=w601, f=w621) -> (s? t:f=w559:bool)
                    "COR_2I 2" <- w559
                    n195 = feedback-in #3(w559) -> ()
                    n196 = feedback #8() -> (w604:bool)
                    n197 = Select(t=FALSE, s="RESET", f=w604) -> (s? t:f=w605:bool)
                    n198 = Select(t=TRUE, s=w602, f=w625) -> (s? t:f=w560:bool)
                    "COR_1I 2" <- w560
                    n199 = feedback-in #4(w560) -> ()
                    n200 = Select(t=TRUE, s=w599, f=w613) -> (s? t:f=w557:bool)
                    "TAM_GI 2" <- w557
                    n201 = feedback-in #5(w557) -> ()
                    n202 = Select(t=TRUE, s=w603, f=w629) -> (s? t:f=w561:bool)
                    "MATERIAL\nMETÁLICO" <- w561
                    n203 = feedback-in #6(w561) -> ()
                    n204 = Select(t=TRUE, s=w598, f=w609) -> (s? t:f=w556:bool)
                    "TAM_MI 2" <- w556
                    n205 = feedback-in #7(w556) -> ()
                    n206 = Select(t=TRUE, s=w597, f=w605) -> (s? t:f=w555:bool)
                    "TAM_PI 2" <- w555
                    n207 = feedback-in #8(w555) -> ()
                  }
                }
                n208 = feedback #9() -> (w360:i32)
                "Numeric" <- w360
                n209 = Select(t=w360, s=w343, f=w348) -> (s? t:f=w361:i32)
                n210 = feedback-in #9(w361) -> ()
                n211 = local read "POS_4 2"() -> (w362:bool)
                n212 = local read "POS_1 2"() -> (w365:bool)
                n213 = local read "POS_2 2"() -> (w364:bool)
                n214 = local read "POS_3 2"() -> (w363:bool)
                n215 = feedback #10() -> (w366:dbl)  [unwired: 1 in]
                n216 = Select(t=4.0, s=w362, f=w366) -> (s? t:f=w368:dbl)
                n217 = Select(t=3.0, s=w363, f=w368) -> (s? t:f=w369:dbl)
                n218 = Select(t=2.0, s=w364, f=w369) -> (s? t:f=w370:dbl)
                n219 = Select(t=1.0, s=w365, f=w370) -> (s? t:f=w367:dbl)
                n220 = feedback-in #10(w367) -> ()
                n221 = local write "POS_ATUAL"(w366) -> ()
                n222 = Less?(x=w348, y=2) -> (x < y?=w355:bool)
                n223 = local write "RESET"(w355) -> ()
                n224 = local read "MATERIAL\nMETÁLICO"() -> (w486:bool)
                n225 = local read "MATERIAL\nMETÁLICO"() -> (w535:bool)
                n226 = local read "TAM_MI 2"() -> (w464:bool)
                n227 = local read "TAM_GI 2"() -> (w438:bool)
                n228 = local read "TAM_PI 2"() -> (w463:bool)
                n229 = local read "COR_1I 2"() -> (w467:bool)
                n230 = local read "COR_2I 2"() -> (w466:bool)
                n231 = local read "COR_3I 2"() -> (w465:bool)
                n232 = Compound Arithmetic op=AND(w467, invert w486) -> (w510:bool)
                n233 = local read "MATERIAL\nMETÁLICO"() -> (w401:bool)
                n234 = local read "TAM_MI 2"() -> (w396:bool)
                n235 = local read "TAM_GI 2"() -> (w397:bool)
                n236 = local read "TAM_PI 2"() -> (w395:bool)
                n237 = Select(t=609.0, s=w535, f=600.0) -> (s? t:f=→"COD_M":dbl)
                n238 = local read "COR_1I 2"() -> (w400:bool)
                n239 = local read "COR_2I 2"() -> (w399:bool)
                n240 = local read "COR_3I 2"() -> (w398:bool)
                n241 = Compound Arithmetic op=AND(w438, invert w486) -> (w498:bool)
                n242 = Compound Arithmetic op=AND(w466, invert w486) -> (w508:bool)
                n243 = Compound Arithmetic op=AND(w397, w400, invert w401) -> (w437:bool)
                n244 = Compound Arithmetic op=AND(w464, invert w438, invert w486) -> (w496:bool)
                n245 = Compound Arithmetic op=AND(w401, w400, w397) -> (w419:bool)
                n246 = Compound Arithmetic op=AND(w465, invert w486) -> (w506:bool)
                n247 = local read "COR_1I 2"() -> (w532:bool)
                n248 = local read "COR_2I 2"() -> (w530:bool)
                n249 = local read "COR_3I 2"() -> (w528:bool)
                n250 = Compound Arithmetic op=AND(w463, invert w464, invert w438, invert w486) -> (w494:bool)
                n251 = Compound Arithmetic op=AND(w396, invert w397, w400, invert w401) -> (w435:bool)
                n252 = feedback #11() -> (w440:dbl)  [unwired: 1 in]
                n253 = Select(t=100.0, s=w510, f=w440) -> (s? t:f=w445:dbl)
                n254 = Select(t=103.0, s=w508, f=w445) -> (s? t:f=w444:dbl)
                n255 = Select(t=106.0, s=w506, f=w444) -> (s? t:f=w443:dbl)
                n256 = Compound Arithmetic op=AND(w401, w400, invert w397, w396) -> (w409:bool)
                n257 = Compound Arithmetic op=AND(w467, w486) -> (w504:bool)
                n258 = Select(t=109.0, s=w504, f=w443) -> (s? t:f=w442:dbl)
                n259 = Compound Arithmetic op=AND(w438, w486) -> (w492:bool)
                n260 = Compound Arithmetic op=AND(w395, invert w396, invert w397, w400, invert w401) -> (w433:bool)
                n261 = feedback #12() -> (w523:dbl)  [unwired: 1 in]
                "COD_C" <- w523
                n262 = Select(t=1006.0, s=w528, f=w523) -> (s? t:f=w526:dbl)
                n263 = Select(t=1003.0, s=w530, f=w526) -> (s? t:f=w525:dbl)
                n264 = Select(t=1000.0, s=w532, f=w525) -> (s? t:f=w524:dbl)
                n265 = feedback-in #12(w524) -> ()
                n266 = Compound Arithmetic op=AND(w401, w400, invert w397, invert w396, w395) -> (w408:bool)
                n267 = Compound Arithmetic op=AND(w466, w486) -> (w502:bool)
                n268 = Select(t=112.0, s=w502, f=w442) -> (s? t:f=w441:dbl)
                n269 = Compound Arithmetic op=AND(w464, invert w438, w486) -> (w490:bool)
                n270 = Compound Arithmetic op=AND(w397, w399, invert w401) -> (w431:bool)
                n271 = Compound Arithmetic op=AND(w465, w486) -> (w500:bool)
                n272 = Compound Arithmetic op=AND(w401, w399, w397) -> (w407:bool)
                n273 = Select(t=115.0, s=w500, f=w441) -> (s? t:f=w439:dbl)
                "COD_MC" <- w439
                n274 = feedback-in #11(w439) -> ()
                n275 = local read "TAM_MI 2"() -> (w517:bool)
                n276 = local read "TAM_GI 2"() -> (w516:bool)
                n277 = local read "TAM_PI 2"() -> (w518:bool)
                n278 = Compound Arithmetic op=AND(w463, invert w464, invert w438, w486) -> (w488:bool)
                n279 = Compound Arithmetic op=AND(w396, invert w397, w399, invert w401) -> (w429:bool)
                n280 = Compound Arithmetic op=AND(invert w516, w517) -> (w519:bool)
                n281 = feedback #13() -> (w449:dbl)  [unwired: 1 in]
                "COD_MT" <- w449
                n282 = Select(t=501.0, s=w498, f=w449) -> (s? t:f=w462:dbl)
                n283 = Select(t=502.0, s=w496, f=w462) -> (s? t:f=w461:dbl)
                n284 = Select(t=503.0, s=w494, f=w461) -> (s? t:f=w460:dbl)
                n285 = Select(t=510.0, s=w492, f=w460) -> (s? t:f=w459:dbl)
                n286 = Select(t=511.0, s=w490, f=w459) -> (s? t:f=w458:dbl)
                n287 = Select(t=512.0, s=w488, f=w458) -> (s? t:f=w457:dbl)
                n288 = feedback-in #13(w457) -> ()
                n289 = Compound Arithmetic op=AND(w401, w399, invert w397, w396) -> (w406:bool)
                n290 = Compound Arithmetic op=AND(invert w516, invert w517, w518) -> (w515:bool)
                n291 = feedback #14() -> (w447:dbl)  [unwired: 1 in]
                n292 = Compound Arithmetic op=AND(w395, invert w396, invert w397, w399, invert w401) -> (w427:bool)
                n293 = feedback #15() -> (w511:dbl)  [unwired: 1 in]
                "COD_T" <- w511
                n294 = Select(t=1403.0, s=w515, f=w511) -> (s? t:f=w514:dbl)
                n295 = Select(t=1402.0, s=w519, f=w514) -> (s? t:f=w513:dbl)
                n296 = Select(t=1401.0, s=w516, f=w513) -> (s? t:f=w512:dbl)
                n297 = feedback-in #15(w512) -> ()
                n298 = Compound Arithmetic op=AND(w438, w467) -> (w485:bool)
                n299 = Compound Arithmetic op=AND(w401, w399, invert w397, invert w396, w395) -> (w405:bool)
                n300 = Compound Arithmetic op=AND(w466, invert w438, invert w464, w463) -> (w475:bool)
                n301 = Compound Arithmetic op=AND(w464, invert w438, w467) -> (w483:bool)
                n302 = Select(t=906.0, s=w475, f=w447) -> (s? t:f=w456:dbl)
                n303 = Compound Arithmetic op=AND(w397, w398, invert w401) -> (w425:bool)
                n304 = Compound Arithmetic op=AND(w401, w398, w397) -> (w404:bool)
                n305 = Compound Arithmetic op=AND(w465, w438) -> (w473:bool)
                n306 = Select(t=907.0, s=w473, f=w456) -> (s? t:f=w455:dbl)
                n307 = Compound Arithmetic op=AND(w463, invert w464, invert w438, w467) -> (w481:bool)
                n308 = Compound Arithmetic op=AND(w396, invert w397, w398, invert w401) -> (w423:bool)
                n309 = local read "Numeric"() -> (w359:i32)
                n310 = Compound Arithmetic op=AND(w401, w398, invert w397, w396) -> (w403:bool)
                n311 = Compound Arithmetic op=AND(w465, invert w438, w464) -> (w471:bool)
                n312 = Select(t=908.0, s=w471, f=w455) -> (s? t:f=w454:dbl)
                n313 = Compound Arithmetic op=AND(w438, w466) -> (w479:bool)
                n314 = Add(x=w359, y=5) -> (x+y=w357:i32)
                n315 = Compound Arithmetic op=AND(w395, invert w396, invert w397, w398, invert w401) -> (w421:bool)
                n316 = Equal?(x=w357, y=w348) -> (x = y?=w356:bool)
                n317 = Compound Arithmetic op=AND(w465, invert w438, invert w464, w463) -> (w469:bool)
                n318 = Compound Arithmetic op=AND(w401, w398, invert w397, invert w396, w395) -> (w402:bool)
                n319 = local read "MANUAL"() -> (w375:bool)
                n320 = Compound Arithmetic op=AND(w464, invert w438, w466) -> (w477:bool)
                n321 = Select(t=909.0, s=w469, f=w454) -> (s? t:f=w446:dbl)
                "COD_CT" <- w446
                n322 = Select(t=901.0, s=w485, f=w446) -> (s? t:f=w453:dbl)
                n323 = Select(t=902.0, s=w483, f=w453) -> (s? t:f=w452:dbl)
                n324 = Select(t=903.0, s=w481, f=w452) -> (s? t:f=w451:dbl)
                n325 = Select(t=904.0, s=w479, f=w451) -> (s? t:f=w450:dbl)
                n326 = Less?(x=w348, y=2) -> (x < y?=w349:bool)
                n327 = feedback #16() -> (w376:dbl)  [unwired: 1 in]
                "CODIGO\nPEÇA" <- w376
                n328 = Select(t=1.0, s=w437, f=w376) -> (s? t:f=w394:dbl)
                n329 = Select(t=2.0, s=w435, f=w394) -> (s? t:f=w393:dbl)
                n330 = Select(t=3.0, s=w433, f=w393) -> (s? t:f=w392:dbl)
                n331 = Select(t=4.0, s=w431, f=w392) -> (s? t:f=w391:dbl)
                n332 = Select(t=5.0, s=w429, f=w391) -> (s? t:f=w390:dbl)
                n333 = Select(t=6.0, s=w427, f=w390) -> (s? t:f=w389:dbl)
                n334 = Select(t=7.0, s=w425, f=w389) -> (s? t:f=w388:dbl)
                n335 = Select(t=8.0, s=w423, f=w388) -> (s? t:f=w387:dbl)
                n336 = Select(t=9.0, s=w421, f=w387) -> (s? t:f=w378:dbl)
                n337 = Select(t=10.0, s=w419, f=w378) -> (s? t:f=w386:dbl)
                n338 = Select(t=11.0, s=w409, f=w386) -> (s? t:f=w385:dbl)
                n339 = Select(t=12.0, s=w408, f=w385) -> (s? t:f=w384:dbl)
                n340 = Select(t=13.0, s=w407, f=w384) -> (s? t:f=w383:dbl)
                n341 = Select(t=14.0, s=w406, f=w383) -> (s? t:f=w382:dbl)
                n342 = Select(t=15.0, s=w405, f=w382) -> (s? t:f=w381:dbl)
                n343 = Select(t=16.0, s=w404, f=w381) -> (s? t:f=w380:dbl)
                n344 = Select(t=17.0, s=w403, f=w380) -> (s? t:f=w379:dbl)
                n345 = Select(t=18.0, s=w402, f=w379) -> (s? t:f=w377:dbl)
                n346 = feedback-in #16(w377) -> ()
                n347 = Select(t=905.0, s=w477, f=w450) -> (s? t:f=w448:dbl)
                n348 = feedback-in #14(w448) -> ()
                n349 = Not(x=w349) -> (.not. x?=w351:bool)
                n350 = Or(x=w375, y=w356) -> (x .or. y?=w353:bool)
                n351 = And(x=w353, y=w351) -> (x .and. y?=w352:bool)
                "Numeric 2" <- w348
              }
              n352 = while {
                i -> [w255]
                stop <- w260 stop-if-true
                n353 = feedback #17() -> (w261:dbl)  [unwired: 1 in]
                "CONT_1" <- w261
                n354 = Equal?(x=w261, y=7.0) -> (x = y?=w286:bool)
                n355 = Increment(x=w261) -> (x+1=w283:dbl)
                n356 = Equal?(x=w261, y=0.0) -> (x = y?=w277:bool)
                n357 = Equal?(x=w261, y=2.0) -> (x = y?=w265:bool)
                n358 = Equal?(x=w261, y=4.0) -> (x = y?=w267:bool)
                n359 = Equal?(x=w261, y=6.0) -> (x = y?=w266:bool)
                n360 = Select(t=0.0, s=w286, f=w283) -> (s? t:f=w285:dbl)
                n361 = Select(t=TRUE, s=w277, f=FALSE) -> (s? t:f=→"1":bool)
                n362 = Select(t=TRUE, s=w267, f=FALSE) -> (s? t:f=→"3":bool)
                n363 = Select(t=TRUE, s=w265, f=FALSE) -> (s? t:f=→"2":bool)
                n364 = feedback-in #17(w285) -> ()
                n365 = Select(t=TRUE, s=w266, f=FALSE) -> (s? t:f=→"4":bool)
                n366 = case shown="6" w261 {
                  frame 0, Default {
                    n367 = Insert Into Array(array=bool[] [], index=0, new element #1=FALSE, new element #2=TRUE, new element #3=FALSE) -> (w287:bool[])
                    n368 = call "DAQ Assistant5"("data"=w287) -> ()  [unwired: 17 in, 2 out]
                    n369 = Wait (ms)(milliseconds to wait=u32 5) -> ()  [unwired: 1 out]
                  }
                  frame 1 {
                    n370 = Insert Into Array(array=bool[] [], index=0, new element #1=FALSE, new element #2=TRUE, new element #3=TRUE) -> (w294:bool[])
                    n371 = call "DAQ Assistant6"("data"=w294) -> ()  [unwired: 17 in, 2 out]
                    n372 = Wait (ms)(milliseconds to wait=u32 1) -> ()  [unwired: 1 out]
                  }
                  frame 2 {
                    n373 = Insert Into Array(array=bool[] [], index=0, new element #1=FALSE, new element #2=TRUE, new element #3=TRUE) -> (w301:bool[])
                    n374 = call "DAQ Assistant7"("data"=w301) -> ()  [unwired: 17 in, 2 out]
                    n375 = Wait (ms)(milliseconds to wait=u32 5) -> ()  [unwired: 1 out]
                  }
                  frame 3 {
                    n376 = Insert Into Array(array=bool[] [], index=0, new element #1=TRUE, new element #2=FALSE, new element #3=TRUE) -> (w308:bool[])
                    n377 = call "DAQ Assistant8"("data"=w308) -> ()  [unwired: 17 in, 2 out]
                    n378 = Wait (ms)(milliseconds to wait=u32 1) -> ()  [unwired: 1 out]
                  }
                  frame 4 {
                    n379 = Insert Into Array(array=bool[] [], index=0, new element #1=TRUE, new element #2=FALSE, new element #3=TRUE) -> (w315:bool[])
                    n380 = call "DAQ Assistant9"("data"=w315) -> ()  [unwired: 17 in, 2 out]
                    n381 = Wait (ms)(milliseconds to wait=u32 5) -> ()  [unwired: 1 out]
                  }
                  frame 5 {
                    n382 = Insert Into Array(array=bool[] [], index=0, new element #1=TRUE, new element #2=FALSE, new element #3=FALSE) -> (w322:bool[])
                    n383 = call "DAQ Assistant10"("data"=w322) -> ()  [unwired: 17 in, 2 out]
                    n384 = Wait (ms)(milliseconds to wait=u32 1) -> ()  [unwired: 1 out]
                  }
                  frame 6 {
                    n385 = Insert Into Array(array=bool[] [], index=0, new element #1=TRUE, new element #2=FALSE, new element #3=FALSE) -> (w329:bool[])
                    n386 = call "DAQ Assistant11"("data"=w329) -> ()  [unwired: 17 in, 2 out]
                    n387 = Wait (ms)(milliseconds to wait=u32 100) -> ()  [unwired: 1 out]
                  }
                  frame 7 {
                    n388 = Insert Into Array(array=bool[] [], index=0, new element #1=FALSE, new element #2=TRUE, new element #3=FALSE) -> (w336:bool[])
                    n389 = call "DAQ Assistant12"("data"=w336) -> ()  [unwired: 17 in, 2 out]
                    n390 = Wait (ms)(milliseconds to wait=u32 20) -> ()  [unwired: 1 out]
                  }
                }
                n391 = Greater?(x=w255, y=3) -> (0:w257:bool)
                n392 = local read "TAM_PI 2"() -> (w258:bool)
                n393 = local read "MANUAL"() -> (w259:bool)
                n394 = And(x=w258, y=w257) -> (x .and. y?=w256:bool)
                n395 = Or(x=w259, y=w256) -> (x .or. y?=w260:bool)
              }
            }
            frame "POSICIONAMENTO HASTE" {
              # "LOOP 3 DE ENDEREÇAMENTO"
              n396 = while {
                i -> [w654]
                stop <- w650 stop-if-true
                # "LÓGICA DO POSIONADOR"
                # "DIREITA = T\nESQUERDA = F"
                # "AQUISIÇÃO POSIÇAO FUTURA"
                # "AQUISIÇÃO POSIÇAO ATUAL"
                # "QUANDO HOUVER CONFLITO, A PEÇA SERÁ DIRECIONADA PARA O SLOT 4"
                # "VERIFICAÇÃO DE CONFLITO"
                # "QUANDO HOUVER CONFLITO, A PEÇA SERÁ DIRECIONADA PARA O SLOT 4"
                # "QUALQUER PEÇA QUE NAO CORRESPONDE A NENHUM SLOT SERÁ DEPOSITADO NO SLOT 1"
                n397 = local read "4"() -> (w768:bool)
                n398 = Select(t=TRUE, s=w768, f=FALSE) -> (s? t:f=w769:bool)
                n399 = local read "POS_1 2"() -> (w690:bool)
                n400 = local read "POS_2 2"() -> (w689:bool)
                n401 = local read "POS_3 2"() -> (w688:bool)
                n402 = local read "POS_4 2"() -> (w687:bool)
                n403 = case shown="False" w769 {
                  frame False {
                    # "AQUISIÇÃO DADOS SENSORES ARRAY"
                    # "LEITURA"
                    n404 = call "DAQ Assistant25"() -> ("data"=w774:bool[])  [unwired: 17 in, 2 out]
                    n405 = Index Array(array=w774, index=5) -> (element=w778:bool)
                    n406 = Index Array(array=w774, index=3) -> (element=w777:bool)
                    n407 = Index Array(array=w774, index=5) -> (element=w776:bool)
                    n408 = Index Array(array=w774, index=7) -> (element=w775:bool)
                    n409 = local read "3"() -> (w786:bool)
                    n410 = local read "3"() -> (w785:bool)
                    n411 = local read "1"() -> (w784:bool)
                    n412 = local read "1"() -> (w783:bool)
                    n413 = And(x=w786, y=w778) -> (x .and. y?=w773:bool)
                    n414 = And(x=w785, y=w777) -> (x .and. y?=w772:bool)
                    n415 = And(x=w784, y=w776) -> (x .and. y?=w771:bool)
                    n416 = And(x=w783, y=w775) -> (x .and. y?=w770:bool)
                    n417 = local write "POS_1 2"(w773) -> ()
                    n418 = local write "POS_2 2"(w772) -> ()
                    n419 = local write "POS_3 2"(w771) -> ()
                    n420 = local write "POS_4 2"(w770) -> ()
                  }
                  frame True {
                    w790 = FALSE ("new element/subarray")
                    # "ENVIO DE SINAL PARA ATUADORES"
                    # "ESCRITA"
                    n421 = local read "ESQ 2"() -> (w788:bool)
                    n422 = local read "RUN"() -> (w791:bool)
                    n423 = Not(x=w788) -> (.not. x?=w787:bool)
                    n424 = Insert Into Array(array=bool[] [], index=0, new element #1=w787, new element #2=w791, new element #3=w790) -> (w789:bool[])
                    n425 = local write "ESTEIRA RUN"(w790) -> ()
                    n426 = call "DAQ Assistant29"("data"=w789) -> ()  [unwired: 17 in, 2 out]
                  }
                }
                n427 = feedback #18() -> (w658:dbl)  [unwired: 1 in]
                n428 = Select(t=4.0, s=w687, f=w658) -> (s? t:f=w680:dbl)
                n429 = Select(t=3.0, s=w688, f=w680) -> (s? t:f=w681:dbl)
                n430 = Select(t=2.0, s=w689, f=w681) -> (s? t:f=w682:dbl)
                n431 = Select(t=1.0, s=w690, f=w682) -> (s? t:f=w679:dbl)
                n432 = feedback-in #18(w679) -> ()
                n433 = Equal To 0?(x=w658) -> (x = 0?=w660:bool)
                n434 = Select(t=5.0, s=w660, f=w658) -> (s? t:f=→"POS_ATUAL":dbl)
                n435 = local read "SLOT 5"() -> (w670:bool)
                n436 = local read "SLOT 6"() -> (w669:bool)
                n437 = local read "SLOT 7"() -> (w668:bool)
                n438 = local read "SLOT 8"() -> (w667:bool)
                n439 = local read "POS_ATUAL"() -> (w639:dbl)
                n440 = local read "POS_FUT"() -> (w638:dbl)
                n441 = Equal?(x=w639, y=w638) -> (x = y?=w666:bool)
                n442 = Greater?(x=w639, y=w638) -> (0:w640:bool)
                "ESQ 2" <- w640
                n443 = feedback #19() -> (w655:dbl)  [unwired: 1 in]
                n444 = Select(t=4.0, s=w667, f=w655) -> (s? t:f=w672:dbl)
                n445 = Select(t=3.0, s=w668, f=w672) -> (s? t:f=w673:dbl)
                n446 = Select(t=2.0, s=w669, f=w673) -> (s? t:f=w674:dbl)
                n447 = Select(t=1.0, s=w670, f=w674) -> (s? t:f=w671:dbl)
                n448 = feedback-in #19(w671) -> ()
                n449 = Not(x=w666) -> (.not. x?=w665:bool)
                n450 = Not(x=w640) -> (.not. x?=→"DIR 2":bool)
                n451 = Equal To 0?(x=w655) -> (x = 0?=w657:bool)
                n452 = Select(t=6.0, s=w657, f=w655) -> (s? t:f=→"POS_FUT":dbl)
                n453 = local write "RUN"(w665) -> ()
                n454 = local read "CODIGO\nPEÇA"() -> (w733:dbl)
                n455 = local read "COD_C"() -> (w728:dbl)
                n456 = local read "COD_MT"() -> (w731:dbl)
                n457 = local read "COD_CT"() -> (w730:dbl)
                n458 = local read "COD_MC"() -> (w732:dbl)
                n459 = local read "COD_T"() -> (w727:dbl)
                n460 = local read "COD_M"() -> (w729:dbl)
                n461 = local read "COD_S2 2"() -> (w750:dbl)
                n462 = local read "COD_S3 2"() -> (w742:dbl)
                n463 = local read "COD_S1 2"() -> (w765:dbl)
                n464 = local read "COD_S4 2"() -> (w734:dbl)
                n465 = local read "CONFIGURAÇÃO CONFLITANTE 2"() -> (w694:bool)
                n466 = local read "CONFIGURAÇÃO CONFLITANTE 2"() -> (w691:bool)
                n467 = local read "CONFIGURAÇÃO CONFLITANTE 2"() -> (w696:bool)
                n468 = Equal?(x=w765, y=w733) -> (x = y?=w763:bool)
                n469 = Equal?(x=w765, y=w732) -> (x = y?=w759:bool)
                n470 = Equal?(x=w765, y=w731) -> (x = y?=w758:bool)
                n471 = Equal?(x=w765, y=w730) -> (x = y?=w764:bool)
                n472 = Equal?(x=w765, y=w729) -> (x = y?=w760:bool)
                n473 = Equal?(x=w765, y=w728) -> (x = y?=w761:bool)
                n474 = Equal?(x=w765, y=w727) -> (x = y?=w762:bool)
                n475 = Equal?(x=w750, y=w733) -> (x = y?=w756:bool)
                n476 = Equal?(x=w750, y=w732) -> (x = y?=w752:bool)
                n477 = Equal?(x=w750, y=w731) -> (x = y?=w751:bool)
                n478 = Equal?(x=w750, y=w730) -> (x = y?=w757:bool)
                n479 = Equal?(x=w750, y=w729) -> (x = y?=w753:bool)
                n480 = Equal?(x=w750, y=w728) -> (x = y?=w754:bool)
                n481 = Equal?(x=w750, y=w727) -> (x = y?=w755:bool)
                n482 = Equal?(x=w742, y=w733) -> (x = y?=w748:bool)
                n483 = Equal?(x=w742, y=w732) -> (x = y?=w744:bool)
                n484 = Equal?(x=w742, y=w731) -> (x = y?=w743:bool)
                n485 = Equal?(x=w742, y=w730) -> (x = y?=w749:bool)
                n486 = Equal?(x=w742, y=w729) -> (x = y?=w745:bool)
                n487 = Equal?(x=w742, y=w728) -> (x = y?=w746:bool)
                n488 = Equal?(x=w742, y=w727) -> (x = y?=w747:bool)
                n489 = Equal?(x=w734, y=w733) -> (x = y?=w740:bool)
                n490 = Equal?(x=w734, y=w732) -> (x = y?=w736:bool)
                n491 = Equal?(x=w734, y=w731) -> (x = y?=w735:bool)
                n492 = Equal?(x=w734, y=w730) -> (x = y?=w741:bool)
                n493 = Equal?(x=w734, y=w729) -> (x = y?=w737:bool)
                n494 = Equal?(x=w734, y=w728) -> (x = y?=w738:bool)
                n495 = Equal?(x=w734, y=w727) -> (x = y?=w739:bool)
                n496 = Compound Arithmetic op=OR(w763, w759, w758, w764, w760, w761, w762) -> (w698:bool)
                n497 = Compound Arithmetic op=OR(w756, w752, w751, w757, w753, w754, w755) -> (w697:bool)
                n498 = Compound Arithmetic op=OR(w748, w744, w743, w749, w745, w746, w747) -> (w695:bool)
                n499 = Compound Arithmetic op=OR(w740, w736, w735, w741, w737, w738, w739) -> (w711:bool)
                n500 = Compound Arithmetic op=AND(invert w696, w697) -> (→"SLOT 6":bool)
                n501 = Compound Arithmetic op=AND(invert w694, w695) -> (→"SLOT 7":bool)
                n502 = Or(x=w691, y=w711) -> (x .or. y?=→"SLOT 8":bool)
                n503 = Select(t=1.0, s=w711, f=0.0) -> (s? t:f=w715:dbl)
                n504 = Select(t=1.0, s=w695, f=0.0) -> (s? t:f=w716:dbl)
                n505 = Select(t=1.0, s=w697, f=0.0) -> (s? t:f=w717:dbl)
                n506 = Select(t=1.0, s=w698, f=0.0) -> (s? t:f=w718:dbl)
                n507 = local write "PEÇA NO\nSLOT"(FALSE) -> ()
                n508 = local read "CONFIGURAÇÃO CONFLITANTE 2"() -> (w692:bool)
                n509 = Compound Arithmetic op=ADD(w718, w717, w716, w715) -> (w712:dbl)
                n510 = local read "COD_S1 2"() -> (w710:dbl)
                n511 = local read "COD_S2 2"() -> (w709:dbl)
                n512 = local read "COD_S3 2"() -> (w708:dbl)
                n513 = local read "COD_S4 2"() -> (w707:dbl)
                n514 = Equal?(x=0.0, y=w712) -> (x = y?=w644:bool)
                "PEÇA NÃO\nCONFIGURADA" <- w644
                n515 = Or(x=w698, y=w644) -> (x .or. y?=w693:bool)
                n516 = Equal?(x=w710, y=w709) -> (x = y?=w706:bool)
                n517 = Equal?(x=w710, y=w708) -> (x = y?=w705:bool)
                n518 = Equal?(x=w710, y=w707) -> (x = y?=w704:bool)
                n519 = Equal?(x=w709, y=w708) -> (x = y?=w703:bool)
                n520 = Equal?(x=w709, y=w707) -> (x = y?=w702:bool)
                n521 = Equal?(x=w708, y=w707) -> (x = y?=w701:bool)
                n522 = Compound Arithmetic op=AND(invert w692, w693) -> (→"SLOT 5":bool)
                n523 = Greater?(x=w712, y=1.0) -> (0:w700:bool)
                n524 = Compound Arithmetic op=OR(w706, w705, w704, w703, w702, w701) -> (w699:bool)
                n525 = Or(x=w700, y=w699) -> (x .or. y?=→"CONFIGURAÇÃO CONFLITANTE 2":bool)
                n526 = local read "POS_ATUAL"() -> (w664:dbl)
                n527 = local read "MANUAL"() -> (w661:bool)
                n528 = local read "POS_FUT"() -> (w663:dbl)
                n529 = Equal?(x=w664, y=w663) -> (x = y?=w662:bool)
                n530 = Or(x=w661, y=w662) -> (x .or. y?=w651:bool)
                n531 = Greater?(x=w654, y=5) -> (0:w652:bool)
                n532 = And(x=w651, y=w652) -> (x .and. y?=w650:bool)
              }
              n533 = local write "TRANSPORTE"(FALSE) -> ()
              n534 = local write "POSICIONAMENTO"(TRUE) -> ()
              n535 = local write "EM ESPERA"(FALSE) -> ()
              n536 = local write "DEPÓSITO"(FALSE) -> ()
              n537 = while {
                stop <- w796 stop-if-true
                n538 = feedback #20() -> (w819:dbl)  [unwired: 1 in]
                n539 = Equal?(x=w819, y=5.0) -> (x = y?=w814:bool)
                n540 = Increment(x=w819) -> (x+1=w815:dbl)
                n541 = Equal?(x=w819, y=0.0) -> (x = y?=w816:bool)
                n542 = Equal?(x=w819, y=2.0) -> (x = y?=w818:bool)
                n543 = Equal?(x=w819, y=4.0) -> (x = y?=w817:bool)
                n544 = Select(t=0.0, s=w814, f=w815) -> (s? t:f=w802:dbl)
                n545 = Select(t=TRUE, s=w816, f=FALSE) -> (s? t:f=w801:bool)
                n546 = Select(t=TRUE, s=w817, f=FALSE) -> (s? t:f=w799:bool)
                n547 = Select(t=TRUE, s=w818, f=FALSE) -> (s? t:f=w800:bool)
                n548 = feedback-in #20(w802) -> ()
                n549 = local write "1"(w801) -> ()
                n550 = local write "4"(w799) -> ()
                n551 = local write "3"(w800) -> ()
                n552 = case shown="4" w819 {
                  frame 0, Default {
                    n553 = Insert Into Array(array=bool[] [], index=0, new element #1=FALSE, new element #2=TRUE, new element #3=FALSE) -> (w820:bool[])
                    n554 = call "DAQ Assistant13"("data"=w820) -> ()  [unwired: 17 in, 2 out]
                    n555 = Wait (ms)(milliseconds to wait=u32 5) -> ()  [unwired: 1 out]
                  }
                  frame 1 {
                    n556 = Insert Into Array(array=bool[] [], index=0, new element #1=TRUE, new element #2=FALSE, new element #3=TRUE) -> (w827:bool[])
                    n557 = call "DAQ Assistant14"("data"=w827) -> ()  [unwired: 17 in, 2 out]
                    n558 = Wait (ms)(milliseconds to wait=u32 1) -> ()  [unwired: 1 out]
                  }
                  frame 2 {
                    n559 = Insert Into Array(array=bool[] [], index=0, new element #1=TRUE, new element #2=FALSE, new element #3=TRUE) -> (w834:bool[])
                    n560 = call "DAQ Assistant15"("data"=w834) -> ()  [unwired: 17 in, 2 out]
                    n561 = Wait (ms)(milliseconds to wait=u32 5) -> ()  [unwired: 1 out]
                  }
                  frame 3 {
                    n562 = Insert Into Array(array=bool[] [], index=0, new element #1=TRUE, new element #2=FALSE, new element #3=FALSE) -> (w841:bool[])
                    n563 = call "DAQ Assistant16"("data"=w841) -> ()  [unwired: 17 in, 2 out]
                    n564 = Wait (ms)(milliseconds to wait=u32 1) -> ()  [unwired: 1 out]
                  }
                  frame 4 {
                    n565 = Insert Into Array(array=bool[] [], index=0, new element #1=TRUE, new element #2=FALSE, new element #3=FALSE) -> (w848:bool[])
                    n566 = call "DAQ Assistant17"("data"=w848) -> ()  [unwired: 17 in, 2 out]
                    n567 = Wait (ms)(milliseconds to wait=u32 120) -> ()  [unwired: 1 out]
                  }
                  frame 5 {
                    n568 = Insert Into Array(array=bool[] [], index=0, new element #1=FALSE, new element #2=TRUE, new element #3=FALSE) -> (w855:bool[])
                    n569 = call "DAQ Assistant18"("data"=w855) -> ()  [unwired: 17 in, 2 out]
                    n570 = Wait (ms)(milliseconds to wait=u32 5) -> ()  [unwired: 1 out]
                  }
                }
                n571 = local read "POS_ATUAL"() -> (w797:dbl)
                n572 = local read "POS_FUT"() -> (w798:dbl)
                n573 = local read "MANUAL"() -> (w794:bool)
                n574 = Equal?(x=w797, y=w798) -> (x = y?=w795:bool)
                n575 = Or(x=w794, y=w795) -> (x .or. y?=w796:bool)
              }
            }
            frame "DEPOSITO HASTE" {
              # "DEPOSITO PEÇA NO SLOT"
              # "LOOP 4 DE ENDEREÇAMENTO"
              n576 = while {
                stop <- w871 stop-if-true
                n577 = local read "4"() -> (w868:bool)
                n578 = case shown="False" w868 {
                  frame False {
                    # "LEITURA"
                    n579 = call "DAQ Assistant26"() -> ("data"=w876:bool[])  [unwired: 17 in, 2 out]
                    n580 = Index Array(array=w876, index=5) -> (element=w874:bool)
                    n581 = local read "2"() -> (w877:bool)
                    n582 = Not(x=w874) -> (.not. x?=w873:bool)
                    n583 = And(x=w877, y=w873) -> (x .and. y?=w875:bool)
                    n584 = feedback #21() -> (w872:bool)
                    "PEÇA NO\nSLOT" <- w872
                    n585 = Select(t=TRUE, s=w875, f=w872) -> (s? t:f=w880:bool)
                    n586 = feedback-in #21(w880) -> ()
                  }
                  frame True {
                    w882 = TRUE
                    # "ESCRITA"
                    n587 = Insert Into Array(array=bool[] [], index=0, new element #1=FALSE, new element #2=FALSE, new element #3=w882) -> (w881:bool[])
                    n588 = local write "ESTEIRA RUN"(w882) -> ()
                    n589 = call "DAQ Assistant30"("data"=w881) -> ()  [unwired: 17 in, 2 out]
                  }
                }
                n590 = local read "PEÇA NO\nSLOT"() -> (w870:bool)
                n591 = local read "MANUAL"() -> (w869:bool)
                n592 = Or(x=w869, y=w870) -> (x .or. y?=w871:bool)
              }
              n593 = local write "POSICIONAMENTO"(FALSE) -> ()
              n594 = local write "TRANSPORTE"(FALSE) -> ()
              n595 = local write "EM ESPERA"(FALSE) -> ()
              n596 = local write "DEPÓSITO"(TRUE) -> ()
              n597 = while {
                stop <- w892 stop-if-true
                n598 = feedback #22() -> (w889:dbl)  [unwired: 1 in]
                n599 = Equal?(x=w889, y=3.0) -> (x = y?=w907:bool)
                n600 = Increment(x=w889) -> (x+1=w904:dbl)
                n601 = Equal?(x=w889, y=0.0) -> (x = y?=w900:bool)
                n602 = Equal?(x=w889, y=2.0) -> (x = y?=w895:bool)
                n603 = Select(t=0.0, s=w907, f=w904) -> (s? t:f=w906:dbl)
                n604 = Select(t=TRUE, s=w900, f=FALSE) -> (s? t:f=w894:bool)
                n605 = Select(t=TRUE, s=w895, f=FALSE) -> (s? t:f=w893:bool)
                n606 = feedback-in #22(w906) -> ()
                n607 = local write "2"(w894) -> ()
                n608 = local write "4"(w893) -> ()
                n609 = local write "1"(FALSE ("1")) -> ()
                n610 = local write "3"(FALSE ("3")) -> ()
                n611 = case shown="3" w889 {
                  frame 3 {
                    n612 = Insert Into Array(array=bool[] [], index=0, new element #1=FALSE, new element #2=TRUE, new element #3=TRUE) -> (w908:bool[])
                    n613 = call "DAQ Assistant19"("data"=w908) -> ()  [unwired: 17 in, 2 out]
                    n614 = Wait (ms)(milliseconds to wait=u32 1) -> ()  [unwired: 1 out]
                  }
                  frame 0, Default {
                    n615 = Insert Into Array(array=bool[] [], index=0, new element #1=FALSE, new element #2=TRUE, new element #3=TRUE) -> (w915:bool[])
                    n616 = call "DAQ Assistant20"("data"=w915) -> ()  [unwired: 17 in, 2 out]
                    n617 = Wait (ms)(milliseconds to wait=u32 2) -> ()  [unwired: 1 out]
                  }
                  frame 1 {
                    n618 = Insert Into Array(array=bool[] [], index=0, new element #1=TRUE, new element #2=FALSE, new element #3=FALSE) -> (w922:bool[])
                    n619 = call "DAQ Assistant21"("data"=w922) -> ()  [unwired: 17 in, 2 out]
                    n620 = Wait (ms)(milliseconds to wait=u32 1) -> ()  [unwired: 1 out]
                  }
                  frame 2 {
                    n621 = Insert Into Array(array=bool[] [], index=0, new element #1=TRUE, new element #2=FALSE, new element #3=FALSE) -> (w929:bool[])
                    n622 = call "DAQ Assistant22"("data"=w929) -> ()  [unwired: 17 in, 2 out]
                    n623 = Wait (ms)(milliseconds to wait=u32 80) -> ()  [unwired: 1 out]
                  }
                }
                n624 = local read "PEÇA NO\nSLOT"() -> (w891:bool)
                n625 = local read "MANUAL"() -> (w890:bool)
                n626 = Or(x=w890, y=w891) -> (x .or. y?=w892:bool)
              }
              n627 = local write "PEÇA NA\nESTEIRA"(FALSE ("PEE_I")) -> ()
            }
          }
          n628 = local read "PEÇA NO\nSLOT"() -> (w9:bool)
          n629 = local read "MANUAL"() -> (w10:bool)
          n630 = Or(x=w9, y=w10) -> (x .or. y?=w8:bool)
        }
      }
      frame True {
        n631 = while {
          stop <- w938 stop-if-true
          n632 = Insert Into Array(array=bool[] [], index=0, new element #1=TRUE, new element #2=FALSE, new element #3=FALSE) -> (w940:bool[])
          n633 = call "DAQ Assistant32"("data"=w940) -> ()  [unwired: 17 in, 2 out]
          n634 = Insert Into Array(array=bool[] [], index=0, new element #1="SENTIDO", new element #2="RUN", new element #3="ESTEIRA") -> (w946:bool[])
          n635 = local write "ESTEIRA RUN"("ESTEIRA") -> ()
          n636 = local write "RUN"("RUN") -> ()
          n637 = call "DAQ Assistant31"("data"=w946) -> ()  [unwired: 17 in, 2 out]
          n638 = local read "AUTOMÁTICO"() -> (w938:bool)
        }
      }
    }
    n639 = local read "PEÇA NO\nSLOT"() -> (w4:bool)
  }
